vi "Verification.vi"(1 "appended array 2":string[][](array[string])) -> (0 "Array":i32[][](array[numeric]))   [LabVIEW 2019]
panel:
  in  "stop 2":bool
  in  "Blank Button 48":bool
  in  "Blank Button 47":bool
  in  "Blank Button 46":bool
  in  "Blank Button 45":bool
  in  "Blank Button 44":bool
  in  "Blank Button 43":bool
  in  "Blank Button 42":bool
  in  "Blank Button 41":bool
  in  "Color Box 45":u32(colorbox)
  in  "Color Box 46":u32(colorbox)
  in  "Color Box 48":u32(colorbox)
  in  "Color Box 43":u32(colorbox)
  in  "Color Box 41":u32(colorbox)
  in  "Color Box 42":u32(colorbox)
  in  "Color Box 44":u32(colorbox)
  in  "Color Box 47":u32(colorbox)
  in  "Blank Button 40":bool
  in  "Blank Button 39":bool
  in  "Color Box 40":u32(colorbox)
  in  "Color Box 39":u32(colorbox)
  in  "Blank Button 38":bool
  in  "Blank Button 37":bool
  in  "Color Box 38":u32(colorbox)
  in  "Color Box 37":u32(colorbox)
  in  "Blank Button 36":bool
  in  "Blank Button 35":bool
  in  "Color Box 36":u32(colorbox)
  in  "Color Box 35":u32(colorbox)
  in  "Blank Button 34":bool
  in  "Blank Button 33":bool
  in  "Color Box 34":u32(colorbox)
  in  "Color Box 33":u32(colorbox)
  in  "Blank Button 32":bool
  in  "Blank Button 31":bool
  in  "Color Box 32":u32(colorbox)
  in  "Color Box 31":u32(colorbox)
  in  "Blank Button 30":bool
  in  "Blank Button 29":bool
  in  "Color Box 30":u32(colorbox)
  in  "Color Box 29":u32(colorbox)
  in  "Blank Button 28":bool
  in  "Blank Button 27":bool
  in  "Color Box 28":u32(colorbox)
  in  "Color Box 27":u32(colorbox)
  in  "Blank Button 26":bool
  in  "Blank Button 25":bool
  in  "Color Box 26":u32(colorbox)
  in  "Color Box 25":u32(colorbox)
  in  "Blank Button 24":bool
  in  "Blank Button 23":bool
  in  "Blank Button 22":bool
  in  "Blank Button 21":bool
  in  "Blank Button 20":bool
  in  "Blank Button 19":bool
  in  "Blank Button 18":bool
  in  "Blank Button 17":bool
  in  "Color Box 24":u32(colorbox)
  in  "Color Box 22":u32(colorbox)
  in  "Color Box 21":u32(colorbox)
  in  "Color Box 19":u32(colorbox)
  in  "Color Box 23":u32(colorbox)
  in  "Color Box 18":u32(colorbox)
  in  "Color Box 17":u32(colorbox)
  in  "Color Box 20":u32(colorbox)
  in  "Blank Button 16":bool
  in  "Blank Button 15":bool
  in  "Blank Button 14":bool
  in  "Blank Button 13":bool
  in  "Blank Button 12":bool
  in  "Blank Button 11":bool
  in  "Blank Button 10":bool
  in  "Blank Button 9":bool
  in  "Color Box 16":u32(colorbox)
  in  "Color Box 14":u32(colorbox)
  in  "Color Box 11":u32(colorbox)
  in  "Color Box 13":u32(colorbox)
  in  "Color Box 9":u32(colorbox)
  in  "Color Box 15":u32(colorbox)
  in  "Color Box 12":u32(colorbox)
  in  "Color Box 10":u32(colorbox)
  in  "Blank Button 8":bool
  in  "Blank Button 7":bool
  in  "Blank Button 6":bool
  in  "Blank Button 5":bool
  in  "Blank Button 2":bool
  in  "Blank Button":bool
  in  "Color Box 2":u32(colorbox)
  in  "Color Box":u32(colorbox)
  in  "Blank Button 4":bool
  in  "Blank Button 3":bool
  in  "Color Box 4":u32(colorbox)
  in  "Color Box 3":u32(colorbox)
  in  "Color Box 8":u32(colorbox)
  in  "Color Box 5":u32(colorbox)
  in  "Color Box 6":u32(colorbox)
  in  "Color Box 7":u32(colorbox)
  in  "stop":bool
  in  "Blanc":dbl
  in  "Vert":dbl
  in  "Bleu":dbl
  in  "Orange":dbl
  in  "Jaune":dbl
  in  "Rouge":dbl
  # "Vérification des couleurs"
  # "W"
  # "R"
  # "B"
  # "G"
  # "Y"
  # "O"
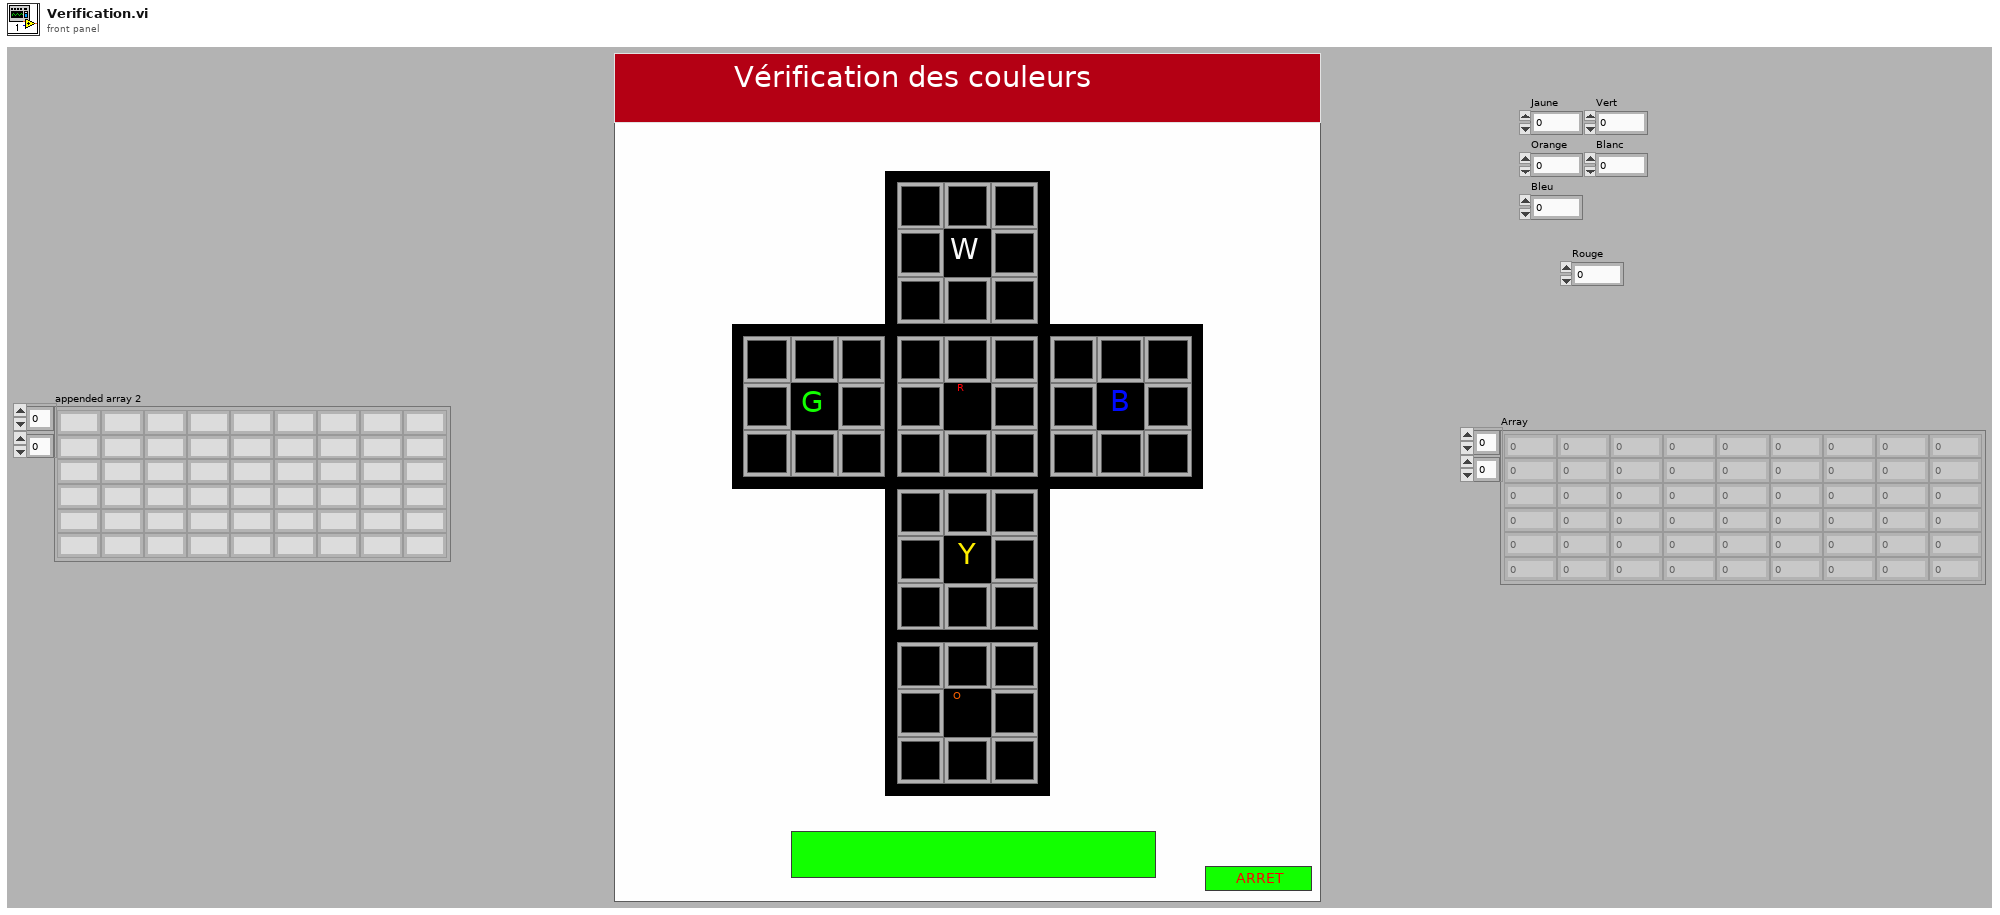
[diagram p1: front panel]
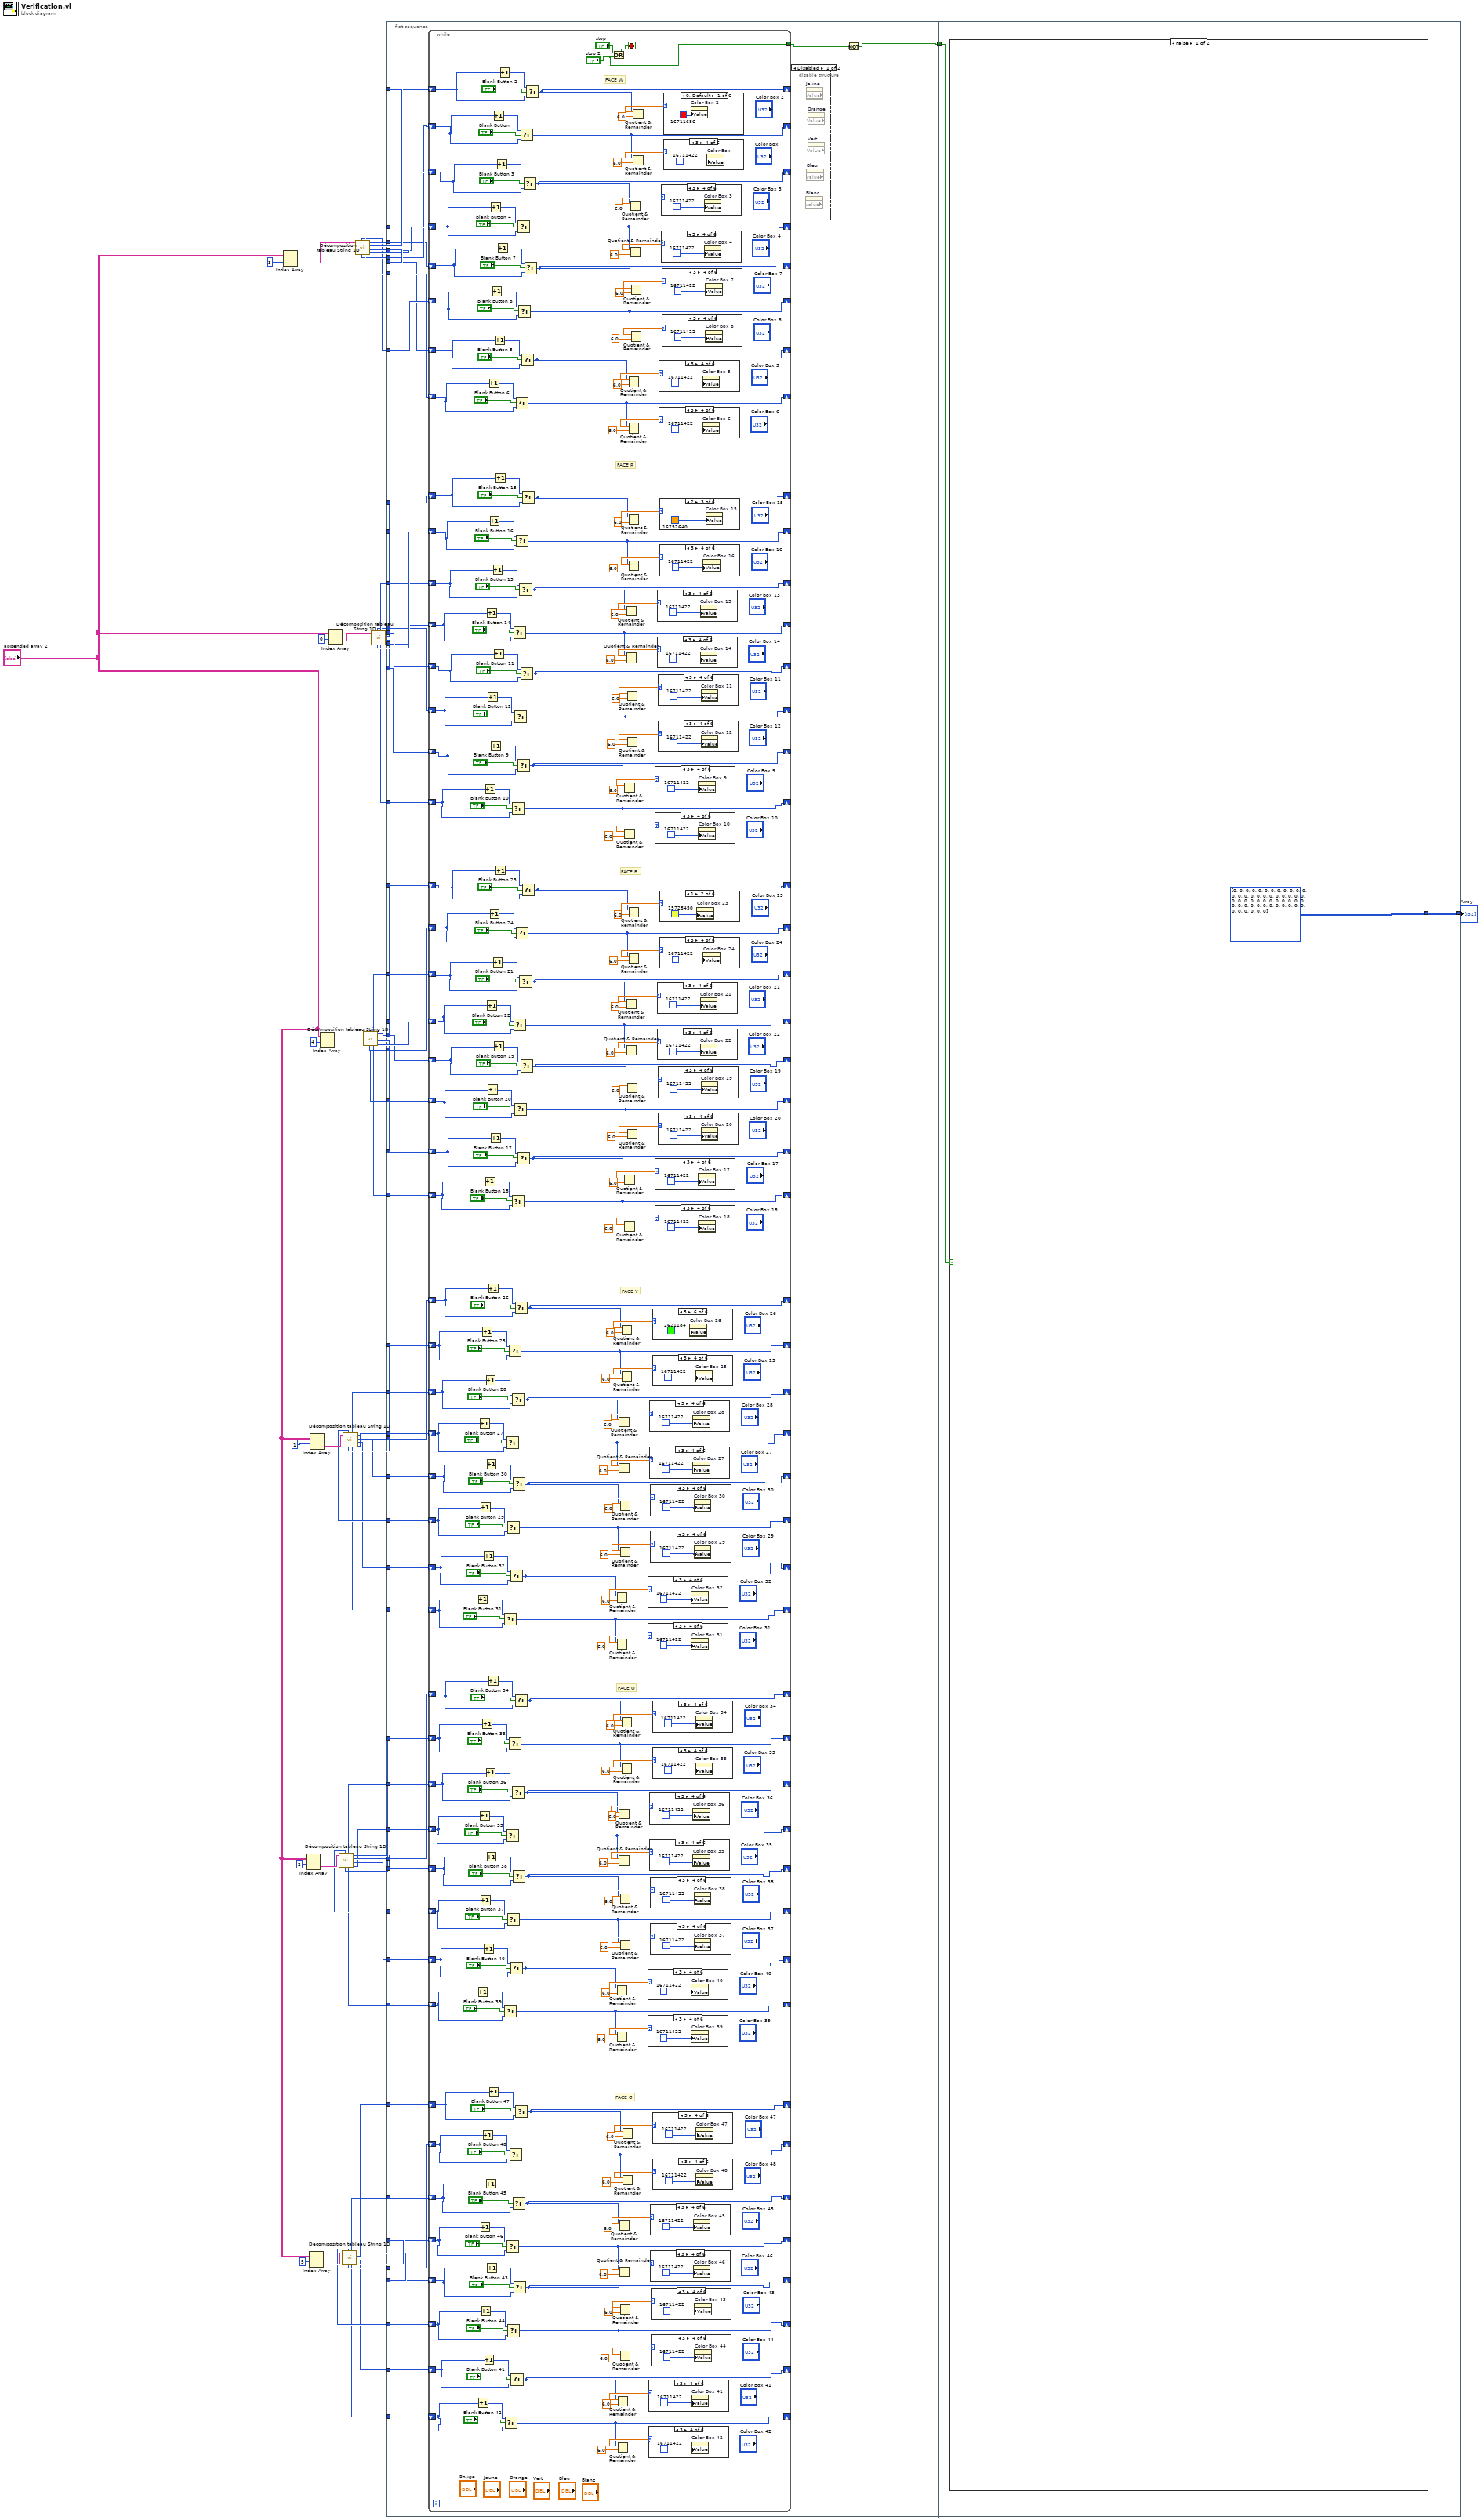
[diagram p0: block diagram]
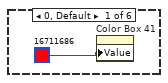
[diagram p3: hidden frame]
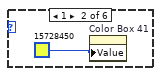
[diagram p4: hidden frame]
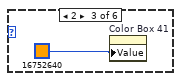
[diagram p5: hidden frame]
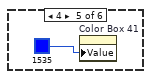
[diagram p6: hidden frame]
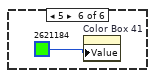
[diagram p7: hidden frame]
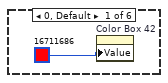
[diagram p8: hidden frame]
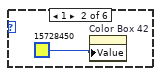
[diagram p9: hidden frame]
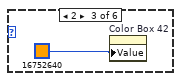
[diagram p10: hidden frame]
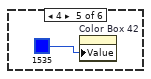
[diagram p11: hidden frame]
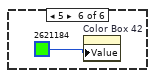
[diagram p12: hidden frame]
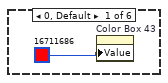
[diagram p13: hidden frame]
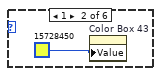
[diagram p14: hidden frame]
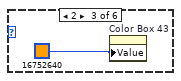
[diagram p15: hidden frame]
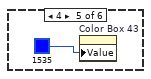
[diagram p16: hidden frame]
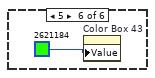
[diagram p17: hidden frame]
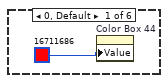
[diagram p18: hidden frame]
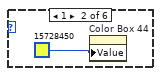
[diagram p19: hidden frame]
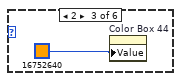
[diagram p20: hidden frame]
diagram:
  n1 = Index Array(array="appended array 2", index (row)=3) -> (element=w62:string[])  [unwired: 1 in]
  n2 = Index Array(array="appended array 2", index (row)=2) -> (element=w38:string[])  [unwired: 1 in]
  n3 = Index Array(array="appended array 2", index (row)=5) -> (element=w39:string[])  [unwired: 1 in]
  n4 = Index Array(array="appended array 2", index (row)=1) -> (element=w37:string[])  [unwired: 1 in]
  n5 = Index Array(array="appended array 2", index (row)=4) -> (element=w42:string[])  [unwired: 1 in]
  n6 = Index Array(array="appended array 2", index (row)=0) -> (element=w53:string[])  [unwired: 1 in]
  n7 = call "Décomposition tableau String 1D.vi"("appended array in"=w38) -> ("7"=w23:i32, "6"=w20:i32, "4"=w26:i32, "3"=w22:i32, "8"=w19:i32, "2"=w24:i32, "9"=w25:i32, "1"=w21:i32)  [unwired: 3 in]
  n8 = call "Décomposition tableau String 1D.vi"("appended array in"=w39) -> ("7"=w31:i32, "6"=w28:i32, "4"=w34:i32, "3"=w30:i32, "8"=w27:i32, "2"=w32:i32, "9"=w33:i32, "1"=w29:i32)  [unwired: 3 in]
  n9 = call "Décomposition tableau String 1D.vi"("appended array in"=w37) -> ("7"=w15:i32, "6"=w12:i32, "4"=w18:i32, "3"=w14:i32, "8"=w11:i32, "2"=w16:i32, "9"=w17:i32, "1"=w13:i32)  [unwired: 3 in]
  n10 = call "Décomposition tableau String 1D.vi"("appended array in"=w62) -> ("7"=w58:i32, "6"=w59:i32, "4"=w55:i32, "3"=w60:i32, "8"=w57:i32, "2"=w61:i32, "9"=w56:i32, "1"=w52:i32)  [unwired: 3 in]
  n11 = call "Décomposition tableau String 1D.vi"("appended array in"=w42) -> ("7"=w7:i32, "6"=w4:i32, "4"=w10:i32, "3"=w6:i32, "8"=w3:i32, "2"=w8:i32, "9"=w9:i32, "1"=w5:i32)  [unwired: 3 in]
  n12 = call "Décomposition tableau String 1D.vi"("appended array in"=w53) -> ("7"=w48:i32, "6"=w45:i32, "4"=w50:i32, "3"=w47:i32, "8"=w44:i32, "2"=w51:i32, "9"=w49:i32, "1"=w46:i32)  [unwired: 3 in]
  n13 = flat-sequence {
    tunnel: w61 -> [w113]
    tunnel: w60 -> [w109]
    tunnel: w58 -> [w112]
    tunnel: w57 -> [w111]
    tunnel: w56 -> [w110]
    tunnel: w55 -> [w64]
    tunnel: w52 -> [w108]
    tunnel: w59 -> [w107]
    tunnel: w44 -> [w106]
    tunnel: w46 -> [w105]
    tunnel: w50 -> [w104]
    tunnel: w49 -> [w103]
    tunnel: w47 -> [w102]
    tunnel: w48 -> [w101]
    tunnel: w51 -> [w100]
    tunnel: w45 -> [w99]
    tunnel: w34 -> [w98]
    tunnel: w33 -> [w97]
    tunnel: w32 -> [w96]
    tunnel: w31 -> [w95]
    tunnel: w30 -> [w94]
    tunnel: w29 -> [w93]
    tunnel: w28 -> [w92]
    tunnel: w27 -> [w91]
    tunnel: w26 -> [w90]
    tunnel: w25 -> [w89]
    tunnel: w24 -> [w88]
    tunnel: w23 -> [w87]
    tunnel: w22 -> [w86]
    tunnel: w21 -> [w85]
    tunnel: w20 -> [w84]
    tunnel: w19 -> [w83]
    tunnel: w18 -> [w82]
    tunnel: w17 -> [w81]
    tunnel: w16 -> [w80]
    tunnel: w15 -> [w79]
    tunnel: w14 -> [w78]
    tunnel: w13 -> [w77]
    tunnel: w12 -> [w76]
    tunnel: w11 -> [w75]
    tunnel: w10 -> [w74]
    tunnel: w9 -> [w73]
    tunnel: w8 -> [w72]
    tunnel: w7 -> [w71]
    tunnel: w6 -> [w70]
    tunnel: w5 -> [w69]
    tunnel: w4 -> [w68]
    tunnel: w3 -> [w67]
    tunnel: [w65] -> w1
    tunnel: [w694] -> w2
    tunnel: w1 -> [w693]
    frame #0 {
      n14 = while {
        shift-right: [w398] -> _
        shift-left: w64 -> [w395]
        shift-right: [w396] -> _
        shift-left: w110 -> [w402]
        shift-right: [w383] -> _
        shift-left: w113 -> [w384]
        shift-right: [w381] -> _
        shift-left: w112 -> [w382]
        shift-right: [w362] -> _
        shift-left: w109 -> [w357]
        shift-right: [w361] -> _
        shift-left: w108 -> [w358]
        shift-right: [w360] -> _
        shift-left: w107 -> [w363]
        shift-right: [w359] -> _
        shift-left: w111 -> [w364]
        shift-right: [w323] -> _
        shift-left: w104 -> [w324]
        shift-right: [w322] -> _
        shift-left: w103 -> [w315]
        shift-right: [w321] -> _
        shift-left: w100 -> [w314]
        shift-right: [w320] -> _
        shift-left: w101 -> [w313]
        shift-right: [w319] -> _
        shift-left: w102 -> [w312]
        shift-right: [w318] -> _
        shift-left: w105 -> [w311]
        shift-right: [w317] -> _
        shift-left: w99 -> [w310]
        shift-right: [w316] -> _
        shift-left: w106 -> [w309]
        shift-right: [w276] -> _
        shift-left: w74 -> [w268]
        shift-right: [w275] -> _
        shift-left: w73 -> [w267]
        shift-right: [w274] -> _
        shift-left: w72 -> [w266]
        shift-right: [w273] -> _
        shift-left: w71 -> [w265]
        shift-right: [w272] -> _
        shift-left: w70 -> [w264]
        shift-right: [w271] -> _
        shift-left: w69 -> [w263]
        shift-right: [w270] -> _
        shift-left: w68 -> [w262]
        shift-right: [w269] -> _
        shift-left: w67 -> [w261]
        shift-right: [w174] -> _
        shift-left: w82 -> [w169]
        shift-right: [w173] -> _
        shift-left: w81 -> [w170]
        shift-right: [w172] -> _
        shift-left: w80 -> [w171]
        shift-right: [w175] -> _
        shift-left: w79 -> [w168]
        shift-right: [w176] -> _
        shift-left: w78 -> [w167]
        shift-right: [w177] -> _
        shift-left: w77 -> [w166]
        shift-right: [w178] -> _
        shift-left: w76 -> [w165]
        shift-right: [w179] -> _
        shift-left: w75 -> [w180]
        shift-right: [w195] -> _
        shift-left: w90 -> [w196]
        shift-right: [w194] -> _
        shift-left: w89 -> [w187]
        shift-right: [w193] -> _
        shift-left: w88 -> [w186]
        shift-right: [w192] -> _
        shift-left: w87 -> [w183]
        shift-right: [w191] -> _
        shift-left: w86 -> [w185]
        shift-right: [w190] -> _
        shift-left: w85 -> [w184]
        shift-right: [w189] -> _
        shift-left: w84 -> [w182]
        shift-right: [w188] -> _
        shift-left: w83 -> [w181]
        shift-right: [w132] -> _
        shift-left: w98 -> [w130]
        shift-right: [w129] -> _
        shift-left: w97 -> [w131]
        shift-right: [w128] -> _
        shift-left: w96 -> [w117]
        shift-right: [w127] -> _
        shift-left: w95 -> [w118]
        shift-right: [w126] -> _
        shift-left: w94 -> [w119]
        shift-right: [w125] -> _
        shift-left: w93 -> [w120]
        shift-right: [w124] -> _
        shift-left: w92 -> [w121]
        shift-right: [w123] -> _
        shift-left: w91 -> [w122]
        tunnel: ["stop 2"] -> w66
        stop <- w116 stop-if-true
        # "FACE G"
        # "FACE O"
        # "FACE Y"
        # "FACE B"
        # "FACE R"
        # "FACE W"
        n15 = Increment(x=w180) -> (x+1=w246:i32)
        n16 = Increment(x=w181) -> (x+1=w211:i32)
        n17 = Increment(x=w122) -> (x+1=w150:i32)
        n18 = Increment(x=w168) -> (x+1=w243:i32)
        n19 = Increment(x=w183) -> (x+1=w214:i32)
        n20 = Increment(x=w118) -> (x+1=w147:i32)
        n21 = Increment(x=w166) -> (x+1=w259:i32)
        n22 = Increment(x=w184) -> (x+1=w198:i32)
        n23 = Increment(x=w120) -> (x+1=w163:i32)
        n24 = Increment(x=w170) -> (x+1=w230:i32)
        n25 = Increment(x=w187) -> (x+1=w227:i32)
        n26 = Increment(x=w131) -> (x+1=w134:i32)
        n27 = Increment(x=w165) -> (x+1=w245:i32)
        n28 = Increment(x=w182) -> (x+1=w212:i32)
        n29 = Increment(x=w121) -> (x+1=w149:i32)
        n30 = Increment(x=w309) -> (x+1=w342:i32)
        n31 = Increment(x=w261) -> (x+1=w291:i32)
        n32 = Increment(x=w171) -> (x+1=w244:i32)
        n33 = Increment(x=w186) -> (x+1=w213:i32)
        n34 = Increment(x=w117) -> (x+1=w148:i32)
        n35 = Increment(x=w167) -> (x+1=w260:i32)
        n36 = Increment(x=w185) -> (x+1=w197:i32)
        n37 = Increment(x=w313) -> (x+1=w339:i32)
        n38 = Increment(x=w265) -> (x+1=w294:i32)
        n39 = Increment(x=w119) -> (x+1=w164:i32)
        n40 = Increment(x=w311) -> (x+1=w355:i32)
        n41 = Increment(x=w263) -> (x+1=w278:i32)
        n42 = Increment(x=w169) -> (x+1=w229:i32)
        n43 = Increment(x=w196) -> (x+1=w228:i32)
        n44 = Increment(x=w130) -> (x+1=w133:i32)
        n45 = Increment(x=w364) -> (x+1=w379:i32)
        n46 = Increment(x=w315) -> (x+1=w326:i32)
        n47 = Increment(x=w267) -> (x+1=w307:i32)
        n48 = Increment(x=w382) -> (x+1=w386:i32)
        n49 = Increment(x=w310) -> (x+1=w341:i32)
        n50 = Increment(x=w262) -> (x+1=w292:i32)
        n51 = Increment(x=w358) -> (x+1=w366:i32)
        n52 = Increment(x=w314) -> (x+1=w340:i32)
        n53 = Increment(x=w266) -> (x+1=w293:i32)
        n54 = Increment(x=w402) -> (x+1=w403:i32)
        n55 = Increment(x=w312) -> (x+1=w356:i32)
        n56 = Increment(x=w264) -> (x+1=w277:i32)
        n57 = Increment(x=w363) -> (x+1=w380:i32)
        n58 = Increment(x=w324) -> (x+1=w325:i32)
        n59 = Increment(x=w268) -> (x+1=w308:i32)
        n60 = Increment(x=w384) -> (x+1=w385:i32)
        n61 = Increment(x=w357) -> (x+1=w365:i32)
        n62 = Increment(x=w395) -> (x+1=w404:i32)
        n63 = Select(t=w246, s="Blank Button 31", f=w180) -> (s? t:f=w179:i32)
        n64 = Select(t=w211, s="Blank Button 39", f=w181) -> (s? t:f=w188:i32)
        n65 = Select(t=w150, s="Blank Button 42", f=w122) -> (s? t:f=w123:i32)
        n66 = Select(t=w243, s="Blank Button 27", f=w168) -> (s? t:f=w175:i32)
        n67 = Select(t=w214, s="Blank Button 35", f=w183) -> (s? t:f=w192:i32)
        n68 = Select(t=w147, s="Blank Button 46", f=w118) -> (s? t:f=w127:i32)
        n69 = Select(t=w259, s="Blank Button 29", f=w166) -> (s? t:f=w177:i32)
        n70 = Select(t=w198, s="Blank Button 37", f=w184) -> (s? t:f=w190:i32)
        n71 = Select(t=w163, s="Blank Button 44", f=w120) -> (s? t:f=w125:i32)
        n72 = Select(t=w230, s="Blank Button 25", f=w170) -> (s? t:f=w173:i32)
        n73 = Select(t=w227, s="Blank Button 33", f=w187) -> (s? t:f=w194:i32)
        n74 = Select(t=w134, s="Blank Button 48", f=w131) -> (s? t:f=w129:i32)
        n75 = Select(t=w245, s="Blank Button 32", f=w165) -> (s? t:f=w178:i32)
        n76 = Select(t=w212, s="Blank Button 40", f=w182) -> (s? t:f=w189:i32)
        n77 = Select(t=w149, s="Blank Button 41", f=w121) -> (s? t:f=w124:i32)
        n78 = Select(t=w342, s="Blank Button 10", f=w309) -> (s? t:f=w316:i32)
        n79 = Select(t=w291, s="Blank Button 18", f=w261) -> (s? t:f=w269:i32)
        n80 = Select(t=w244, s="Blank Button 28", f=w171) -> (s? t:f=w172:i32)
        n81 = Select(t=w213, s="Blank Button 36", f=w186) -> (s? t:f=w193:i32)
        n82 = Select(t=w148, s="Blank Button 45", f=w117) -> (s? t:f=w128:i32)
        n83 = Select(t=w260, s="Blank Button 30", f=w167) -> (s? t:f=w176:i32)
        n84 = Select(t=w197, s="Blank Button 38", f=w185) -> (s? t:f=w191:i32)
        n85 = Select(t=w339, s="Blank Button 14", f=w313) -> (s? t:f=w320:i32)
        n86 = Select(t=w294, s="Blank Button 22", f=w265) -> (s? t:f=w273:i32)
        n87 = Select(t=w164, s="Blank Button 43", f=w119) -> (s? t:f=w126:i32)
        n88 = Select(t=w355, s="Blank Button 12", f=w311) -> (s? t:f=w318:i32)
        n89 = Select(t=w278, s="Blank Button 20", f=w263) -> (s? t:f=w271:i32)
        n90 = Select(t=w229, s="Blank Button 26", f=w169) -> (s? t:f=w174:i32)
        n91 = Select(t=w228, s="Blank Button 34", f=w196) -> (s? t:f=w195:i32)
        n92 = Select(t=w133, s="Blank Button 47", f=w130) -> (s? t:f=w132:i32)
        n93 = Select(t=w379, s="Blank Button 6", f=w364) -> (s? t:f=w359:i32)
        n94 = Select(t=w326, s="Blank Button 16", f=w315) -> (s? t:f=w322:i32)
        n95 = Select(t=w307, s="Blank Button 24", f=w267) -> (s? t:f=w275:i32)
        n96 = Select(t=w386, s="Blank Button 4", f=w382) -> (s? t:f=w381:i32)
        n97 = Select(t=w341, s="Blank Button 9", f=w310) -> (s? t:f=w317:i32)
        n98 = Select(t=w292, s="Blank Button 17", f=w262) -> (s? t:f=w270:i32)
        n99 = Select(t=w366, s="Blank Button 8", f=w358) -> (s? t:f=w361:i32)
        n100 = Select(t=w340, s="Blank Button 13", f=w314) -> (s? t:f=w321:i32)
        n101 = Select(t=w293, s="Blank Button 21", f=w266) -> (s? t:f=w274:i32)
        n102 = Select(t=w403, s="Blank Button", f=w402) -> (s? t:f=w396:i32)
        n103 = Select(t=w356, s="Blank Button 11", f=w312) -> (s? t:f=w319:i32)
        n104 = Select(t=w277, s="Blank Button 19", f=w264) -> (s? t:f=w272:i32)
        n105 = Select(t=w380, s="Blank Button 5", f=w363) -> (s? t:f=w360:i32)
        n106 = Select(t=w325, s="Blank Button 15", f=w324) -> (s? t:f=w323:i32)
        n107 = Select(t=w308, s="Blank Button 23", f=w268) -> (s? t:f=w276:i32)
        n108 = Select(t=w385, s="Blank Button 3", f=w384) -> (s? t:f=w383:i32)
        n109 = Select(t=w365, s="Blank Button 7", f=w357) -> (s? t:f=w362:i32)
        n110 = Select(t=w404, s="Blank Button 2", f=w395) -> (s? t:f=w398:i32)
        n111 = Or(x="stop", y="stop 2") -> (x .or. y?=w116:bool)
        n112 = Quotient & Remainder(x=w178, y=6.0) -> (x-y*floor(x/y)=w249:dbl)  [unwired: 1 out]
        n113 = Quotient & Remainder(x=w179, y=6.0) -> (x-y*floor(x/y)=w247:dbl)  [unwired: 1 out]
        n114 = Quotient & Remainder(x=w189, y=6.0) -> (x-y*floor(x/y)=w208:dbl)  [unwired: 1 out]
        n115 = Quotient & Remainder(x=w188, y=6.0) -> (x-y*floor(x/y)=w210:dbl)  [unwired: 1 out]
        n116 = Quotient & Remainder(x=w124, y=6.0) -> (x-y*floor(x/y)=w153:dbl)  [unwired: 1 out]
        n117 = Quotient & Remainder(x=w123, y=6.0) -> (x-y*floor(x/y)=w151:dbl)  [unwired: 1 out]
        n118 = Quotient & Remainder(x=w172, y=6.0) -> (x-y*floor(x/y)=w240:dbl)  [unwired: 1 out]
        n119 = Quotient & Remainder(x=w175, y=6.0) -> (x-y*floor(x/y)=w242:dbl)  [unwired: 1 out]
        n120 = Quotient & Remainder(x=w193, y=6.0) -> (x-y*floor(x/y)=w217:dbl)  [unwired: 1 out]
        n121 = Quotient & Remainder(x=w192, y=6.0) -> (x-y*floor(x/y)=w215:dbl)  [unwired: 1 out]
        n122 = Quotient & Remainder(x=w128, y=6.0) -> (x-y*floor(x/y)=w144:dbl)  [unwired: 1 out]
        n123 = Quotient & Remainder(x=w127, y=6.0) -> (x-y*floor(x/y)=w146:dbl)  [unwired: 1 out]
        n124 = Quotient & Remainder(x=w176, y=6.0) -> (x-y*floor(x/y)=w256:dbl)  [unwired: 1 out]
        n125 = Quotient & Remainder(x=w177, y=6.0) -> (x-y*floor(x/y)=w258:dbl)  [unwired: 1 out]
        n126 = Quotient & Remainder(x=w191, y=6.0) -> (x-y*floor(x/y)=w201:dbl)  [unwired: 1 out]
        n127 = Quotient & Remainder(x=w190, y=6.0) -> (x-y*floor(x/y)=w199:dbl)  [unwired: 1 out]
        n128 = Quotient & Remainder(x=w126, y=6.0) -> (x-y*floor(x/y)=w160:dbl)  [unwired: 1 out]
        n129 = Quotient & Remainder(x=w125, y=6.0) -> (x-y*floor(x/y)=w162:dbl)  [unwired: 1 out]
        n130 = Quotient & Remainder(x=w174, y=6.0) -> (x-y*floor(x/y)=w233:dbl)  [unwired: 1 out]
        n131 = Quotient & Remainder(x=w173, y=6.0) -> (x-y*floor(x/y)=w231:dbl)  [unwired: 1 out]
        n132 = Quotient & Remainder(x=w195, y=6.0) -> (x-y*floor(x/y)=w224:dbl)  [unwired: 1 out]
        n133 = Quotient & Remainder(x=w194, y=6.0) -> (x-y*floor(x/y)=w226:dbl)  [unwired: 1 out]
        n134 = Quotient & Remainder(x=w132, y=6.0) -> (x-y*floor(x/y)=w137:dbl)  [unwired: 1 out]
        n135 = Quotient & Remainder(x=w129, y=6.0) -> (x-y*floor(x/y)=w135:dbl)  [unwired: 1 out]
        n136 = Quotient & Remainder(x=w317, y=6.0) -> (x-y*floor(x/y)=w345:dbl)  [unwired: 1 out]
        n137 = Quotient & Remainder(x=w316, y=6.0) -> (x-y*floor(x/y)=w343:dbl)  [unwired: 1 out]
        n138 = Quotient & Remainder(x=w270, y=6.0) -> (x-y*floor(x/y)=w288:dbl)  [unwired: 1 out]
        n139 = Quotient & Remainder(x=w269, y=6.0) -> (x-y*floor(x/y)=w290:dbl)  [unwired: 1 out]
        n140 = Quotient & Remainder(x=w321, y=6.0) -> (x-y*floor(x/y)=w336:dbl)  [unwired: 1 out]
        n141 = Quotient & Remainder(x=w320, y=6.0) -> (x-y*floor(x/y)=w338:dbl)  [unwired: 1 out]
        n142 = Quotient & Remainder(x=w274, y=6.0) -> (x-y*floor(x/y)=w297:dbl)  [unwired: 1 out]
        n143 = Quotient & Remainder(x=w273, y=6.0) -> (x-y*floor(x/y)=w295:dbl)  [unwired: 1 out]
        n144 = Quotient & Remainder(x=w319, y=6.0) -> (x-y*floor(x/y)=w352:dbl)  [unwired: 1 out]
        n145 = Quotient & Remainder(x=w318, y=6.0) -> (x-y*floor(x/y)=w354:dbl)  [unwired: 1 out]
        n146 = Quotient & Remainder(x=w272, y=6.0) -> (x-y*floor(x/y)=w281:dbl)  [unwired: 1 out]
        n147 = Quotient & Remainder(x=w271, y=6.0) -> (x-y*floor(x/y)=w279:dbl)  [unwired: 1 out]
        n148 = Quotient & Remainder(x=w360, y=6.0) -> (x-y*floor(x/y)=w376:dbl)  [unwired: 1 out]
        n149 = Quotient & Remainder(x=w359, y=6.0) -> (x-y*floor(x/y)=w378:dbl)  [unwired: 1 out]
        n150 = Quotient & Remainder(x=w323, y=6.0) -> (x-y*floor(x/y)=w329:dbl)  [unwired: 1 out]
        n151 = Quotient & Remainder(x=w322, y=6.0) -> (x-y*floor(x/y)=w327:dbl)  [unwired: 1 out]
        n152 = Quotient & Remainder(x=w276, y=6.0) -> (x-y*floor(x/y)=w304:dbl)  [unwired: 1 out]
        n153 = Quotient & Remainder(x=w275, y=6.0) -> (x-y*floor(x/y)=w306:dbl)  [unwired: 1 out]
        n154 = Quotient & Remainder(x=w383, y=6.0) -> (x-y*floor(x/y)=w389:dbl)  [unwired: 1 out]
        n155 = Quotient & Remainder(x=w381, y=6.0) -> (x-y*floor(x/y)=w387:dbl)  [unwired: 1 out]
        n156 = Quotient & Remainder(x=w362, y=6.0) -> (x-y*floor(x/y)=w369:dbl)  [unwired: 1 out]
        n157 = Quotient & Remainder(x=w361, y=6.0) -> (x-y*floor(x/y)=w367:dbl)  [unwired: 1 out]
        n158 = Quotient & Remainder(x=w398, y=6.0) -> (x-y*floor(x/y)=w399:dbl)  [unwired: 1 out]
        n159 = Quotient & Remainder(x=w396, y=6.0) -> (x-y*floor(x/y)=w401:dbl)  [unwired: 1 out]
        n160 = case shown="3" w249 {
          frame 0, Default {
            n161 = property on="Color Box 32" class="ColBox"("Value"=u32 16711686 ("Color Box")) -> ()  [unwired: 2 in, 2 out]
          }
          frame 1 {
            n162 = property on="Color Box 32" class="ColBox"("Value"=u32 15728450 ("Color Box")) -> ()  [unwired: 2 in, 2 out]
          }
          frame 2 {
            n163 = property on="Color Box 32" class="ColBox"("Value"=u32 16752640 ("Color Box")) -> ()  [unwired: 2 in, 2 out]
          }
          frame 3 {
            n164 = property on="Color Box 32" class="ColBox"("Value"=u32 16711422 ("Color Box")) -> ()  [unwired: 2 in, 2 out]
          }
          frame 4 {
            n165 = property on="Color Box 32" class="ColBox"("Value"=u32 1535 ("Color Box")) -> ()  [unwired: 2 in, 2 out]
          }
          frame 5 {
            n166 = property on="Color Box 32" class="ColBox"("Value"=u32 2621184 ("Color Box")) -> ()  [unwired: 2 in, 2 out]
          }
        }
        n167 = case shown="3" w247 {
          frame 0, Default {
            n168 = property on="Color Box 31" class="ColBox"("Value"=u32 16711686 ("Color Box")) -> ()  [unwired: 2 in, 2 out]
          }
          frame 1 {
            n169 = property on="Color Box 31" class="ColBox"("Value"=u32 15728450 ("Color Box")) -> ()  [unwired: 2 in, 2 out]
          }
          frame 2 {
            n170 = property on="Color Box 31" class="ColBox"("Value"=u32 16752640 ("Color Box")) -> ()  [unwired: 2 in, 2 out]
          }
          frame 3 {
            n171 = property on="Color Box 31" class="ColBox"("Value"=u32 16711422 ("Color Box")) -> ()  [unwired: 2 in, 2 out]
          }
          frame 4 {
            n172 = property on="Color Box 31" class="ColBox"("Value"=u32 1535 ("Color Box")) -> ()  [unwired: 2 in, 2 out]
          }
          frame 5 {
            n173 = property on="Color Box 31" class="ColBox"("Value"=u32 2621184 ("Color Box")) -> ()  [unwired: 2 in, 2 out]
          }
        }
        n174 = case shown="3" w208 {
          frame 0, Default {
            n175 = property on="Color Box 40" class="ColBox"("Value"=u32 16711686 ("Color Box")) -> ()  [unwired: 2 in, 2 out]
          }
          frame 1 {
            n176 = property on="Color Box 40" class="ColBox"("Value"=u32 15728450 ("Color Box")) -> ()  [unwired: 2 in, 2 out]
          }
          frame 2 {
            n177 = property on="Color Box 40" class="ColBox"("Value"=u32 16752640 ("Color Box")) -> ()  [unwired: 2 in, 2 out]
          }
          frame 3 {
            n178 = property on="Color Box 40" class="ColBox"("Value"=u32 16711422 ("Color Box")) -> ()  [unwired: 2 in, 2 out]
          }
          frame 4 {
            n179 = property on="Color Box 40" class="ColBox"("Value"=u32 1535 ("Color Box")) -> ()  [unwired: 2 in, 2 out]
          }
          frame 5 {
            n180 = property on="Color Box 40" class="ColBox"("Value"=u32 2621184 ("Color Box")) -> ()  [unwired: 2 in, 2 out]
          }
        }
        n181 = case shown="3" w210 {
          frame 0, Default {
            n182 = property on="Color Box 39" class="ColBox"("Value"=u32 16711686 ("Color Box")) -> ()  [unwired: 2 in, 2 out]
          }
          frame 1 {
            n183 = property on="Color Box 39" class="ColBox"("Value"=u32 15728450 ("Color Box")) -> ()  [unwired: 2 in, 2 out]
          }
          frame 2 {
            n184 = property on="Color Box 39" class="ColBox"("Value"=u32 16752640 ("Color Box")) -> ()  [unwired: 2 in, 2 out]
          }
          frame 3 {
            n185 = property on="Color Box 39" class="ColBox"("Value"=u32 16711422 ("Color Box")) -> ()  [unwired: 2 in, 2 out]
          }
          frame 4 {
            n186 = property on="Color Box 39" class="ColBox"("Value"=u32 1535 ("Color Box")) -> ()  [unwired: 2 in, 2 out]
          }
          frame 5 {
            n187 = property on="Color Box 39" class="ColBox"("Value"=u32 2621184 ("Color Box")) -> ()  [unwired: 2 in, 2 out]
          }
        }
        n188 = case shown="3" w153 {
          frame 0, Default {
            n189 = property on="Color Box 41" class="ColBox"("Value"=u32 16711686 ("Color Box")) -> ()  [unwired: 2 in, 2 out]
          }
          frame 1 {
            n190 = property on="Color Box 41" class="ColBox"("Value"=u32 15728450 ("Color Box")) -> ()  [unwired: 2 in, 2 out]
          }
          frame 2 {
            n191 = property on="Color Box 41" class="ColBox"("Value"=u32 16752640 ("Color Box")) -> ()  [unwired: 2 in, 2 out]
          }
          frame 3 {
            n192 = property on="Color Box 41" class="ColBox"("Value"=u32 16711422 ("Color Box")) -> ()  [unwired: 2 in, 2 out]
          }
          frame 4 {
            n193 = property on="Color Box 41" class="ColBox"("Value"=u32 1535 ("Color Box")) -> ()  [unwired: 2 in, 2 out]
          }
          frame 5 {
            n194 = property on="Color Box 41" class="ColBox"("Value"=u32 2621184 ("Color Box")) -> ()  [unwired: 2 in, 2 out]
          }
        }
        n195 = case shown="3" w151 {
          frame 0, Default {
            n196 = property on="Color Box 42" class="ColBox"("Value"=u32 16711686 ("Color Box")) -> ()  [unwired: 2 in, 2 out]
          }
          frame 1 {
            n197 = property on="Color Box 42" class="ColBox"("Value"=u32 15728450 ("Color Box")) -> ()  [unwired: 2 in, 2 out]
          }
          frame 2 {
            n198 = property on="Color Box 42" class="ColBox"("Value"=u32 16752640 ("Color Box")) -> ()  [unwired: 2 in, 2 out]
          }
          frame 3 {
            n199 = property on="Color Box 42" class="ColBox"("Value"=u32 16711422 ("Color Box")) -> ()  [unwired: 2 in, 2 out]
          }
          frame 4 {
            n200 = property on="Color Box 42" class="ColBox"("Value"=u32 1535 ("Color Box")) -> ()  [unwired: 2 in, 2 out]
          }
          frame 5 {
            n201 = property on="Color Box 42" class="ColBox"("Value"=u32 2621184 ("Color Box")) -> ()  [unwired: 2 in, 2 out]
          }
        }
        n202 = case shown="3" w240 {
          frame 0, Default {
            n203 = property on="Color Box 28" class="ColBox"("Value"=u32 16711686 ("Color Box")) -> ()  [unwired: 2 in, 2 out]
          }
          frame 1 {
            n204 = property on="Color Box 28" class="ColBox"("Value"=u32 15728450 ("Color Box")) -> ()  [unwired: 2 in, 2 out]
          }
          frame 2 {
            n205 = property on="Color Box 28" class="ColBox"("Value"=u32 16752640 ("Color Box")) -> ()  [unwired: 2 in, 2 out]
          }
          frame 3 {
            n206 = property on="Color Box 28" class="ColBox"("Value"=u32 16711422 ("Color Box")) -> ()  [unwired: 2 in, 2 out]
          }
          frame 4 {
            n207 = property on="Color Box 28" class="ColBox"("Value"=u32 1535 ("Color Box")) -> ()  [unwired: 2 in, 2 out]
          }
          frame 5 {
            n208 = property on="Color Box 28" class="ColBox"("Value"=u32 2621184 ("Color Box")) -> ()  [unwired: 2 in, 2 out]
          }
        }
        n209 = case shown="3" w242 {
          frame 0, Default {
            n210 = property on="Color Box 27" class="ColBox"("Value"=u32 16711686 ("Color Box")) -> ()  [unwired: 2 in, 2 out]
          }
          frame 1 {
            n211 = property on="Color Box 27" class="ColBox"("Value"=u32 15728450 ("Color Box")) -> ()  [unwired: 2 in, 2 out]
          }
          frame 2 {
            n212 = property on="Color Box 27" class="ColBox"("Value"=u32 16752640 ("Color Box")) -> ()  [unwired: 2 in, 2 out]
          }
          frame 3 {
            n213 = property on="Color Box 27" class="ColBox"("Value"=u32 16711422 ("Color Box")) -> ()  [unwired: 2 in, 2 out]
          }
          frame 4 {
            n214 = property on="Color Box 27" class="ColBox"("Value"=u32 1535 ("Color Box")) -> ()  [unwired: 2 in, 2 out]
          }
          frame 5 {
            n215 = property on="Color Box 27" class="ColBox"("Value"=u32 2621184 ("Color Box")) -> ()  [unwired: 2 in, 2 out]
          }
        }
        n216 = case shown="3" w217 {
          frame 0, Default {
            n217 = property on="Color Box 36" class="ColBox"("Value"=u32 16711686 ("Color Box")) -> ()  [unwired: 2 in, 2 out]
          }
          frame 1 {
            n218 = property on="Color Box 36" class="ColBox"("Value"=u32 15728450 ("Color Box")) -> ()  [unwired: 2 in, 2 out]
          }
          frame 2 {
            n219 = property on="Color Box 36" class="ColBox"("Value"=u32 16752640 ("Color Box")) -> ()  [unwired: 2 in, 2 out]
          }
          frame 3 {
            n220 = property on="Color Box 36" class="ColBox"("Value"=u32 16711422 ("Color Box")) -> ()  [unwired: 2 in, 2 out]
          }
          frame 4 {
            n221 = property on="Color Box 36" class="ColBox"("Value"=u32 1535 ("Color Box")) -> ()  [unwired: 2 in, 2 out]
          }
          frame 5 {
            n222 = property on="Color Box 36" class="ColBox"("Value"=u32 2621184 ("Color Box")) -> ()  [unwired: 2 in, 2 out]
          }
        }
        n223 = case shown="3" w215 {
          frame 0, Default {
            n224 = property on="Color Box 35" class="ColBox"("Value"=u32 16711686 ("Color Box")) -> ()  [unwired: 2 in, 2 out]
          }
          frame 1 {
            n225 = property on="Color Box 35" class="ColBox"("Value"=u32 15728450 ("Color Box")) -> ()  [unwired: 2 in, 2 out]
          }
          frame 2 {
            n226 = property on="Color Box 35" class="ColBox"("Value"=u32 16752640 ("Color Box")) -> ()  [unwired: 2 in, 2 out]
          }
          frame 3 {
            n227 = property on="Color Box 35" class="ColBox"("Value"=u32 16711422 ("Color Box")) -> ()  [unwired: 2 in, 2 out]
          }
          frame 4 {
            n228 = property on="Color Box 35" class="ColBox"("Value"=u32 1535 ("Color Box")) -> ()  [unwired: 2 in, 2 out]
          }
          frame 5 {
            n229 = property on="Color Box 35" class="ColBox"("Value"=u32 2621184 ("Color Box")) -> ()  [unwired: 2 in, 2 out]
          }
        }
        n230 = case shown="3" w144 {
          frame 0, Default {
            n231 = property on="Color Box 45" class="ColBox"("Value"=u32 16711686 ("Color Box")) -> ()  [unwired: 2 in, 2 out]
          }
          frame 1 {
            n232 = property on="Color Box 45" class="ColBox"("Value"=u32 15728450 ("Color Box")) -> ()  [unwired: 2 in, 2 out]
          }
          frame 2 {
            n233 = property on="Color Box 45" class="ColBox"("Value"=u32 16752640 ("Color Box")) -> ()  [unwired: 2 in, 2 out]
          }
          frame 3 {
            n234 = property on="Color Box 45" class="ColBox"("Value"=u32 16711422 ("Color Box")) -> ()  [unwired: 2 in, 2 out]
          }
          frame 4 {
            n235 = property on="Color Box 45" class="ColBox"("Value"=u32 1535 ("Color Box")) -> ()  [unwired: 2 in, 2 out]
          }
          frame 5 {
            n236 = property on="Color Box 45" class="ColBox"("Value"=u32 2621184 ("Color Box")) -> ()  [unwired: 2 in, 2 out]
          }
        }
        n237 = case shown="3" w146 {
          frame 0, Default {
            n238 = property on="Color Box 46" class="ColBox"("Value"=u32 16711686 ("Color Box")) -> ()  [unwired: 2 in, 2 out]
          }
          frame 1 {
            n239 = property on="Color Box 46" class="ColBox"("Value"=u32 15728450 ("Color Box")) -> ()  [unwired: 2 in, 2 out]
          }
          frame 2 {
            n240 = property on="Color Box 46" class="ColBox"("Value"=u32 16752640 ("Color Box")) -> ()  [unwired: 2 in, 2 out]
          }
          frame 3 {
            n241 = property on="Color Box 46" class="ColBox"("Value"=u32 16711422 ("Color Box")) -> ()  [unwired: 2 in, 2 out]
          }
          frame 4 {
            n242 = property on="Color Box 46" class="ColBox"("Value"=u32 1535 ("Color Box")) -> ()  [unwired: 2 in, 2 out]
          }
          frame 5 {
            n243 = property on="Color Box 46" class="ColBox"("Value"=u32 2621184 ("Color Box")) -> ()  [unwired: 2 in, 2 out]
          }
        }
        n244 = case shown="3" w256 {
          frame 0, Default {
            n245 = property on="Color Box 30" class="ColBox"("Value"=u32 16711686 ("Color Box")) -> ()  [unwired: 2 in, 2 out]
          }
          frame 1 {
            n246 = property on="Color Box 30" class="ColBox"("Value"=u32 15728450 ("Color Box")) -> ()  [unwired: 2 in, 2 out]
          }
          frame 2 {
            n247 = property on="Color Box 30" class="ColBox"("Value"=u32 16752640 ("Color Box")) -> ()  [unwired: 2 in, 2 out]
          }
          frame 3 {
            n248 = property on="Color Box 30" class="ColBox"("Value"=u32 16711422 ("Color Box")) -> ()  [unwired: 2 in, 2 out]
          }
          frame 4 {
            n249 = property on="Color Box 30" class="ColBox"("Value"=u32 1535 ("Color Box")) -> ()  [unwired: 2 in, 2 out]
          }
          frame 5 {
            n250 = property on="Color Box 30" class="ColBox"("Value"=u32 2621184 ("Color Box")) -> ()  [unwired: 2 in, 2 out]
          }
        }
        n251 = case shown="3" w258 {
          frame 0, Default {
            n252 = property on="Color Box 29" class="ColBox"("Value"=u32 16711686 ("Color Box")) -> ()  [unwired: 2 in, 2 out]
          }
          frame 1 {
            n253 = property on="Color Box 29" class="ColBox"("Value"=u32 15728450 ("Color Box")) -> ()  [unwired: 2 in, 2 out]
          }
          frame 2 {
            n254 = property on="Color Box 29" class="ColBox"("Value"=u32 16752640 ("Color Box")) -> ()  [unwired: 2 in, 2 out]
          }
          frame 3 {
            n255 = property on="Color Box 29" class="ColBox"("Value"=u32 16711422 ("Color Box")) -> ()  [unwired: 2 in, 2 out]
          }
          frame 4 {
            n256 = property on="Color Box 29" class="ColBox"("Value"=u32 1535 ("Color Box")) -> ()  [unwired: 2 in, 2 out]
          }
          frame 5 {
            n257 = property on="Color Box 29" class="ColBox"("Value"=u32 2621184 ("Color Box")) -> ()  [unwired: 2 in, 2 out]
          }
        }
        n258 = case shown="3" w201 {
          frame 0, Default {
            n259 = property on="Color Box 38" class="ColBox"("Value"=u32 16711686 ("Color Box")) -> ()  [unwired: 2 in, 2 out]
          }
          frame 1 {
            n260 = property on="Color Box 38" class="ColBox"("Value"=u32 15728450 ("Color Box")) -> ()  [unwired: 2 in, 2 out]
          }
          frame 2 {
            n261 = property on="Color Box 38" class="ColBox"("Value"=u32 16752640 ("Color Box")) -> ()  [unwired: 2 in, 2 out]
          }
          frame 3 {
            n262 = property on="Color Box 38" class="ColBox"("Value"=u32 16711422 ("Color Box")) -> ()  [unwired: 2 in, 2 out]
          }
          frame 4 {
            n263 = property on="Color Box 38" class="ColBox"("Value"=u32 1535 ("Color Box")) -> ()  [unwired: 2 in, 2 out]
          }
          frame 5 {
            n264 = property on="Color Box 38" class="ColBox"("Value"=u32 2621184 ("Color Box")) -> ()  [unwired: 2 in, 2 out]
          }
        }
        n265 = case shown="3" w199 {
          frame 0, Default {
            n266 = property on="Color Box 37" class="ColBox"("Value"=u32 16711686 ("Color Box")) -> ()  [unwired: 2 in, 2 out]
          }
          frame 1 {
            n267 = property on="Color Box 37" class="ColBox"("Value"=u32 15728450 ("Color Box")) -> ()  [unwired: 2 in, 2 out]
          }
          frame 2 {
            n268 = property on="Color Box 37" class="ColBox"("Value"=u32 16752640 ("Color Box")) -> ()  [unwired: 2 in, 2 out]
          }
          frame 3 {
            n269 = property on="Color Box 37" class="ColBox"("Value"=u32 16711422 ("Color Box")) -> ()  [unwired: 2 in, 2 out]
          }
          frame 4 {
            n270 = property on="Color Box 37" class="ColBox"("Value"=u32 1535 ("Color Box")) -> ()  [unwired: 2 in, 2 out]
          }
          frame 5 {
            n271 = property on="Color Box 37" class="ColBox"("Value"=u32 2621184 ("Color Box")) -> ()  [unwired: 2 in, 2 out]
          }
        }
        n272 = case shown="3" w160 {
          frame 0, Default {
            n273 = property on="Color Box 43" class="ColBox"("Value"=u32 16711686 ("Color Box")) -> ()  [unwired: 2 in, 2 out]
          }
          frame 1 {
            n274 = property on="Color Box 43" class="ColBox"("Value"=u32 15728450 ("Color Box")) -> ()  [unwired: 2 in, 2 out]
          }
          frame 2 {
            n275 = property on="Color Box 43" class="ColBox"("Value"=u32 16752640 ("Color Box")) -> ()  [unwired: 2 in, 2 out]
          }
          frame 3 {
            n276 = property on="Color Box 43" class="ColBox"("Value"=u32 16711422 ("Color Box")) -> ()  [unwired: 2 in, 2 out]
          }
          frame 4 {
            n277 = property on="Color Box 43" class="ColBox"("Value"=u32 1535 ("Color Box")) -> ()  [unwired: 2 in, 2 out]
          }
          frame 5 {
            n278 = property on="Color Box 43" class="ColBox"("Value"=u32 2621184 ("Color Box")) -> ()  [unwired: 2 in, 2 out]
          }
        }
        n279 = case shown="3" w162 {
          frame 0, Default {
            n280 = property on="Color Box 44" class="ColBox"("Value"=u32 16711686 ("Color Box")) -> ()  [unwired: 2 in, 2 out]
          }
          frame 1 {
            n281 = property on="Color Box 44" class="ColBox"("Value"=u32 15728450 ("Color Box")) -> ()  [unwired: 2 in, 2 out]
          }
          frame 2 {
            n282 = property on="Color Box 44" class="ColBox"("Value"=u32 16752640 ("Color Box")) -> ()  [unwired: 2 in, 2 out]
          }
          frame 3 {
            n283 = property on="Color Box 44" class="ColBox"("Value"=u32 16711422 ("Color Box")) -> ()  [unwired: 2 in, 2 out]
          }
          frame 4 {
            n284 = property on="Color Box 44" class="ColBox"("Value"=u32 1535 ("Color Box")) -> ()  [unwired: 2 in, 2 out]
          }
          frame 5 {
            n285 = property on="Color Box 44" class="ColBox"("Value"=u32 2621184 ("Color Box")) -> ()  [unwired: 2 in, 2 out]
          }
        }
        n286 = case shown="5" w233 {
          frame 0, Default {
            n287 = property on="Color Box 26" class="ColBox"("Value"=u32 16711686 ("Color Box")) -> ()  [unwired: 2 in, 2 out]
          }
          frame 1 {
            n288 = property on="Color Box 26" class="ColBox"("Value"=u32 15728450 ("Color Box")) -> ()  [unwired: 2 in, 2 out]
          }
          frame 2 {
            n289 = property on="Color Box 26" class="ColBox"("Value"=u32 16752640 ("Color Box")) -> ()  [unwired: 2 in, 2 out]
          }
          frame 3 {
            n290 = property on="Color Box 26" class="ColBox"("Value"=u32 16711422 ("Color Box")) -> ()  [unwired: 2 in, 2 out]
          }
          frame 4 {
            n291 = property on="Color Box 26" class="ColBox"("Value"=u32 1535 ("Color Box")) -> ()  [unwired: 2 in, 2 out]
          }
          frame 5 {
            n292 = property on="Color Box 26" class="ColBox"("Value"=u32 2621184 ("Color Box")) -> ()  [unwired: 2 in, 2 out]
          }
        }
        n293 = case shown="3" w231 {
          frame 0, Default {
            n294 = property on="Color Box 25" class="ColBox"("Value"=u32 16711686 ("Color Box")) -> ()  [unwired: 2 in, 2 out]
          }
          frame 1 {
            n295 = property on="Color Box 25" class="ColBox"("Value"=u32 15728450 ("Color Box")) -> ()  [unwired: 2 in, 2 out]
          }
          frame 2 {
            n296 = property on="Color Box 25" class="ColBox"("Value"=u32 16752640 ("Color Box")) -> ()  [unwired: 2 in, 2 out]
          }
          frame 3 {
            n297 = property on="Color Box 25" class="ColBox"("Value"=u32 16711422 ("Color Box")) -> ()  [unwired: 2 in, 2 out]
          }
          frame 4 {
            n298 = property on="Color Box 25" class="ColBox"("Value"=u32 1535 ("Color Box")) -> ()  [unwired: 2 in, 2 out]
          }
          frame 5 {
            n299 = property on="Color Box 25" class="ColBox"("Value"=u32 2621184 ("Color Box")) -> ()  [unwired: 2 in, 2 out]
          }
        }
        n300 = case shown="3" w224 {
          frame 0, Default {
            n301 = property on="Color Box 34" class="ColBox"("Value"=u32 16711686 ("Color Box")) -> ()  [unwired: 2 in, 2 out]
          }
          frame 1 {
            n302 = property on="Color Box 34" class="ColBox"("Value"=u32 15728450 ("Color Box")) -> ()  [unwired: 2 in, 2 out]
          }
          frame 2 {
            n303 = property on="Color Box 34" class="ColBox"("Value"=u32 16752640 ("Color Box")) -> ()  [unwired: 2 in, 2 out]
          }
          frame 3 {
            n304 = property on="Color Box 34" class="ColBox"("Value"=u32 16711422 ("Color Box")) -> ()  [unwired: 2 in, 2 out]
          }
          frame 4 {
            n305 = property on="Color Box 34" class="ColBox"("Value"=u32 1535 ("Color Box")) -> ()  [unwired: 2 in, 2 out]
          }
          frame 5 {
            n306 = property on="Color Box 34" class="ColBox"("Value"=u32 2621184 ("Color Box")) -> ()  [unwired: 2 in, 2 out]
          }
        }
        n307 = case shown="3" w226 {
          frame 0, Default {
            n308 = property on="Color Box 33" class="ColBox"("Value"=u32 16711686 ("Color Box")) -> ()  [unwired: 2 in, 2 out]
          }
          frame 1 {
            n309 = property on="Color Box 33" class="ColBox"("Value"=u32 15728450 ("Color Box")) -> ()  [unwired: 2 in, 2 out]
          }
          frame 2 {
            n310 = property on="Color Box 33" class="ColBox"("Value"=u32 16752640 ("Color Box")) -> ()  [unwired: 2 in, 2 out]
          }
          frame 3 {
            n311 = property on="Color Box 33" class="ColBox"("Value"=u32 16711422 ("Color Box")) -> ()  [unwired: 2 in, 2 out]
          }
          frame 4 {
            n312 = property on="Color Box 33" class="ColBox"("Value"=u32 1535 ("Color Box")) -> ()  [unwired: 2 in, 2 out]
          }
          frame 5 {
            n313 = property on="Color Box 33" class="ColBox"("Value"=u32 2621184 ("Color Box")) -> ()  [unwired: 2 in, 2 out]
          }
        }
        n314 = case shown="3" w137 {
          frame 0, Default {
            n315 = property on="Color Box 47" class="ColBox"("Value"=u32 16711686 ("Color Box")) -> ()  [unwired: 2 in, 2 out]
          }
          frame 1 {
            n316 = property on="Color Box 47" class="ColBox"("Value"=u32 15728450 ("Color Box")) -> ()  [unwired: 2 in, 2 out]
          }
          frame 2 {
            n317 = property on="Color Box 47" class="ColBox"("Value"=u32 16752640 ("Color Box")) -> ()  [unwired: 2 in, 2 out]
          }
          frame 3 {
            n318 = property on="Color Box 47" class="ColBox"("Value"=u32 16711422 ("Color Box")) -> ()  [unwired: 2 in, 2 out]
          }
          frame 4 {
            n319 = property on="Color Box 47" class="ColBox"("Value"=u32 1535 ("Color Box")) -> ()  [unwired: 2 in, 2 out]
          }
          frame 5 {
            n320 = property on="Color Box 47" class="ColBox"("Value"=u32 2621184 ("Color Box")) -> ()  [unwired: 2 in, 2 out]
          }
        }
        n321 = case shown="3" w135 {
          frame 0, Default {
            n322 = property on="Color Box 48" class="ColBox"("Value"=u32 16711686 ("Color Box")) -> ()  [unwired: 2 in, 2 out]
          }
          frame 1 {
            n323 = property on="Color Box 48" class="ColBox"("Value"=u32 15728450 ("Color Box")) -> ()  [unwired: 2 in, 2 out]
          }
          frame 2 {
            n324 = property on="Color Box 48" class="ColBox"("Value"=u32 16752640 ("Color Box")) -> ()  [unwired: 2 in, 2 out]
          }
          frame 3 {
            n325 = property on="Color Box 48" class="ColBox"("Value"=u32 16711422 ("Color Box")) -> ()  [unwired: 2 in, 2 out]
          }
          frame 4 {
            n326 = property on="Color Box 48" class="ColBox"("Value"=u32 1535 ("Color Box")) -> ()  [unwired: 2 in, 2 out]
          }
          frame 5 {
            n327 = property on="Color Box 48" class="ColBox"("Value"=u32 2621184 ("Color Box")) -> ()  [unwired: 2 in, 2 out]
          }
        }
        n328 = case shown="3" w345 {
          frame 0, Default {
            n329 = property on="Color Box 9" class="ColBox"("Value"=u32 16711686 ("Color Box")) -> ()  [unwired: 2 in, 2 out]
          }
          frame 1 {
            n330 = property on="Color Box 9" class="ColBox"("Value"=u32 15728450 ("Color Box")) -> ()  [unwired: 2 in, 2 out]
          }
          frame 2 {
            n331 = property on="Color Box 9" class="ColBox"("Value"=u32 16752640 ("Color Box")) -> ()  [unwired: 2 in, 2 out]
          }
          frame 3 {
            n332 = property on="Color Box 9" class="ColBox"("Value"=u32 16711422 ("Color Box")) -> ()  [unwired: 2 in, 2 out]
          }
          frame 4 {
            n333 = property on="Color Box 9" class="ColBox"("Value"=u32 1535 ("Color Box")) -> ()  [unwired: 2 in, 2 out]
          }
          frame 5 {
            n334 = property on="Color Box 9" class="ColBox"("Value"=u32 2621184 ("Color Box")) -> ()  [unwired: 2 in, 2 out]
          }
        }
        n335 = case shown="3" w343 {
          frame 0, Default {
            n336 = property on="Color Box 10" class="ColBox"("Value"=u32 16711686 ("Color Box")) -> ()  [unwired: 2 in, 2 out]
          }
          frame 1 {
            n337 = property on="Color Box 10" class="ColBox"("Value"=u32 15728450 ("Color Box")) -> ()  [unwired: 2 in, 2 out]
          }
          frame 2 {
            n338 = property on="Color Box 10" class="ColBox"("Value"=u32 16752640 ("Color Box")) -> ()  [unwired: 2 in, 2 out]
          }
          frame 3 {
            n339 = property on="Color Box 10" class="ColBox"("Value"=u32 16711422 ("Color Box")) -> ()  [unwired: 2 in, 2 out]
          }
          frame 4 {
            n340 = property on="Color Box 10" class="ColBox"("Value"=u32 1535 ("Color Box")) -> ()  [unwired: 2 in, 2 out]
          }
          frame 5 {
            n341 = property on="Color Box 10" class="ColBox"("Value"=u32 2621184 ("Color Box")) -> ()  [unwired: 2 in, 2 out]
          }
        }
        n342 = case shown="3" w288 {
          frame 0, Default {
            n343 = property on="Color Box 17" class="ColBox"("Value"=u32 16711686 ("Color Box")) -> ()  [unwired: 2 in, 2 out]
          }
          frame 1 {
            n344 = property on="Color Box 17" class="ColBox"("Value"=u32 15728450 ("Color Box")) -> ()  [unwired: 2 in, 2 out]
          }
          frame 2 {
            n345 = property on="Color Box 17" class="ColBox"("Value"=u32 16752640 ("Color Box")) -> ()  [unwired: 2 in, 2 out]
          }
          frame 3 {
            n346 = property on="Color Box 17" class="ColBox"("Value"=u32 16711422 ("Color Box")) -> ()  [unwired: 2 in, 2 out]
          }
          frame 4 {
            n347 = property on="Color Box 17" class="ColBox"("Value"=u32 1535 ("Color Box")) -> ()  [unwired: 2 in, 2 out]
          }
          frame 5 {
            n348 = property on="Color Box 17" class="ColBox"("Value"=u32 2621184 ("Color Box")) -> ()  [unwired: 2 in, 2 out]
          }
        }
        n349 = case shown="3" w290 {
          frame 0, Default {
            n350 = property on="Color Box 18" class="ColBox"("Value"=u32 16711686 ("Color Box")) -> ()  [unwired: 2 in, 2 out]
          }
          frame 1 {
            n351 = property on="Color Box 18" class="ColBox"("Value"=u32 15728450 ("Color Box")) -> ()  [unwired: 2 in, 2 out]
          }
          frame 2 {
            n352 = property on="Color Box 18" class="ColBox"("Value"=u32 16752640 ("Color Box")) -> ()  [unwired: 2 in, 2 out]
          }
          frame 3 {
            n353 = property on="Color Box 18" class="ColBox"("Value"=u32 16711422 ("Color Box")) -> ()  [unwired: 2 in, 2 out]
          }
          frame 4 {
            n354 = property on="Color Box 18" class="ColBox"("Value"=u32 1535 ("Color Box")) -> ()  [unwired: 2 in, 2 out]
          }
          frame 5 {
            n355 = property on="Color Box 18" class="ColBox"("Value"=u32 2621184 ("Color Box")) -> ()  [unwired: 2 in, 2 out]
          }
        }
        n356 = case shown="3" w336 {
          frame 0, Default {
            n357 = property on="Color Box 13" class="ColBox"("Value"=u32 16711686 ("Color Box")) -> ()  [unwired: 2 in, 2 out]
          }
          frame 1 {
            n358 = property on="Color Box 13" class="ColBox"("Value"=u32 15728450 ("Color Box")) -> ()  [unwired: 2 in, 2 out]
          }
          frame 2 {
            n359 = property on="Color Box 13" class="ColBox"("Value"=u32 16752640 ("Color Box")) -> ()  [unwired: 2 in, 2 out]
          }
          frame 3 {
            n360 = property on="Color Box 13" class="ColBox"("Value"=u32 16711422 ("Color Box")) -> ()  [unwired: 2 in, 2 out]
          }
          frame 4 {
            n361 = property on="Color Box 13" class="ColBox"("Value"=u32 1535 ("Color Box")) -> ()  [unwired: 2 in, 2 out]
          }
          frame 5 {
            n362 = property on="Color Box 13" class="ColBox"("Value"=u32 2621184 ("Color Box")) -> ()  [unwired: 2 in, 2 out]
          }
        }
        n363 = case shown="3" w338 {
          frame 0, Default {
            n364 = property on="Color Box 14" class="ColBox"("Value"=u32 16711686 ("Color Box")) -> ()  [unwired: 2 in, 2 out]
          }
          frame 1 {
            n365 = property on="Color Box 14" class="ColBox"("Value"=u32 15728450 ("Color Box")) -> ()  [unwired: 2 in, 2 out]
          }
          frame 2 {
            n366 = property on="Color Box 14" class="ColBox"("Value"=u32 16752640 ("Color Box")) -> ()  [unwired: 2 in, 2 out]
          }
          frame 3 {
            n367 = property on="Color Box 14" class="ColBox"("Value"=u32 16711422 ("Color Box")) -> ()  [unwired: 2 in, 2 out]
          }
          frame 4 {
            n368 = property on="Color Box 14" class="ColBox"("Value"=u32 1535 ("Color Box")) -> ()  [unwired: 2 in, 2 out]
          }
          frame 5 {
            n369 = property on="Color Box 14" class="ColBox"("Value"=u32 2621184 ("Color Box")) -> ()  [unwired: 2 in, 2 out]
          }
        }
        n370 = case shown="3" w297 {
          frame 0, Default {
            n371 = property on="Color Box 21" class="ColBox"("Value"=u32 16711686 ("Color Box")) -> ()  [unwired: 2 in, 2 out]
          }
          frame 1 {
            n372 = property on="Color Box 21" class="ColBox"("Value"=u32 15728450 ("Color Box")) -> ()  [unwired: 2 in, 2 out]
          }
          frame 2 {
            n373 = property on="Color Box 21" class="ColBox"("Value"=u32 16752640 ("Color Box")) -> ()  [unwired: 2 in, 2 out]
          }
          frame 3 {
            n374 = property on="Color Box 21" class="ColBox"("Value"=u32 16711422 ("Color Box")) -> ()  [unwired: 2 in, 2 out]
          }
          frame 4 {
            n375 = property on="Color Box 21" class="ColBox"("Value"=u32 1535 ("Color Box")) -> ()  [unwired: 2 in, 2 out]
          }
          frame 5 {
            n376 = property on="Color Box 21" class="ColBox"("Value"=u32 2621184 ("Color Box")) -> ()  [unwired: 2 in, 2 out]
          }
        }
        n377 = case shown="3" w295 {
          frame 0, Default {
            n378 = property on="Color Box 22" class="ColBox"("Value"=u32 16711686 ("Color Box")) -> ()  [unwired: 2 in, 2 out]
          }
          frame 1 {
            n379 = property on="Color Box 22" class="ColBox"("Value"=u32 15728450 ("Color Box")) -> ()  [unwired: 2 in, 2 out]
          }
          frame 2 {
            n380 = property on="Color Box 22" class="ColBox"("Value"=u32 16752640 ("Color Box")) -> ()  [unwired: 2 in, 2 out]
          }
          frame 3 {
            n381 = property on="Color Box 22" class="ColBox"("Value"=u32 16711422 ("Color Box")) -> ()  [unwired: 2 in, 2 out]
          }
          frame 4 {
            n382 = property on="Color Box 22" class="ColBox"("Value"=u32 1535 ("Color Box")) -> ()  [unwired: 2 in, 2 out]
          }
          frame 5 {
            n383 = property on="Color Box 22" class="ColBox"("Value"=u32 2621184 ("Color Box")) -> ()  [unwired: 2 in, 2 out]
          }
        }
        n384 = case shown="3" w352 {
          frame 0, Default {
            n385 = property on="Color Box 11" class="ColBox"("Value"=u32 16711686 ("Color Box")) -> ()  [unwired: 2 in, 2 out]
          }
          frame 1 {
            n386 = property on="Color Box 11" class="ColBox"("Value"=u32 15728450 ("Color Box")) -> ()  [unwired: 2 in, 2 out]
          }
          frame 2 {
            n387 = property on="Color Box 11" class="ColBox"("Value"=u32 16752640 ("Color Box")) -> ()  [unwired: 2 in, 2 out]
          }
          frame 3 {
            n388 = property on="Color Box 11" class="ColBox"("Value"=u32 16711422 ("Color Box")) -> ()  [unwired: 2 in, 2 out]
          }
          frame 4 {
            n389 = property on="Color Box 11" class="ColBox"("Value"=u32 1535 ("Color Box")) -> ()  [unwired: 2 in, 2 out]
          }
          frame 5 {
            n390 = property on="Color Box 11" class="ColBox"("Value"=u32 2621184 ("Color Box")) -> ()  [unwired: 2 in, 2 out]
          }
        }
        n391 = case shown="3" w354 {
          frame 0, Default {
            n392 = property on="Color Box 12" class="ColBox"("Value"=u32 16711686 ("Color Box")) -> ()  [unwired: 2 in, 2 out]
          }
          frame 1 {
            n393 = property on="Color Box 12" class="ColBox"("Value"=u32 15728450 ("Color Box")) -> ()  [unwired: 2 in, 2 out]
          }
          frame 2 {
            n394 = property on="Color Box 12" class="ColBox"("Value"=u32 16752640 ("Color Box")) -> ()  [unwired: 2 in, 2 out]
          }
          frame 3 {
            n395 = property on="Color Box 12" class="ColBox"("Value"=u32 16711422 ("Color Box")) -> ()  [unwired: 2 in, 2 out]
          }
          frame 4 {
            n396 = property on="Color Box 12" class="ColBox"("Value"=u32 1535 ("Color Box")) -> ()  [unwired: 2 in, 2 out]
          }
          frame 5 {
            n397 = property on="Color Box 12" class="ColBox"("Value"=u32 2621184 ("Color Box")) -> ()  [unwired: 2 in, 2 out]
          }
        }
        n398 = case shown="3" w281 {
          frame 0, Default {
            n399 = property on="Color Box 19" class="ColBox"("Value"=u32 16711686 ("Color Box")) -> ()  [unwired: 2 in, 2 out]
          }
          frame 1 {
            n400 = property on="Color Box 19" class="ColBox"("Value"=u32 15728450 ("Color Box")) -> ()  [unwired: 2 in, 2 out]
          }
          frame 2 {
            n401 = property on="Color Box 19" class="ColBox"("Value"=u32 16752640 ("Color Box")) -> ()  [unwired: 2 in, 2 out]
          }
          frame 3 {
            n402 = property on="Color Box 19" class="ColBox"("Value"=u32 16711422 ("Color Box")) -> ()  [unwired: 2 in, 2 out]
          }
          frame 4 {
            n403 = property on="Color Box 19" class="ColBox"("Value"=u32 1535 ("Color Box")) -> ()  [unwired: 2 in, 2 out]
          }
          frame 5 {
            n404 = property on="Color Box 19" class="ColBox"("Value"=u32 2621184 ("Color Box")) -> ()  [unwired: 2 in, 2 out]
          }
        }
        n405 = case shown="3" w279 {
          frame 0, Default {
            n406 = property on="Color Box 20" class="ColBox"("Value"=u32 16711686 ("Color Box")) -> ()  [unwired: 2 in, 2 out]
          }
          frame 1 {
            n407 = property on="Color Box 20" class="ColBox"("Value"=u32 15728450 ("Color Box")) -> ()  [unwired: 2 in, 2 out]
          }
          frame 2 {
            n408 = property on="Color Box 20" class="ColBox"("Value"=u32 16752640 ("Color Box")) -> ()  [unwired: 2 in, 2 out]
          }
          frame 3 {
            n409 = property on="Color Box 20" class="ColBox"("Value"=u32 16711422 ("Color Box")) -> ()  [unwired: 2 in, 2 out]
          }
          frame 4 {
            n410 = property on="Color Box 20" class="ColBox"("Value"=u32 1535 ("Color Box")) -> ()  [unwired: 2 in, 2 out]
          }
          frame 5 {
            n411 = property on="Color Box 20" class="ColBox"("Value"=u32 2621184 ("Color Box")) -> ()  [unwired: 2 in, 2 out]
          }
        }
        n412 = case shown="3" w376 {
          frame 0, Default {
            n413 = property on="Color Box 5" class="ColBox"("Value"=u32 16711686 ("Color Box")) -> ()  [unwired: 2 in, 2 out]
          }
          frame 1 {
            n414 = property on="Color Box 5" class="ColBox"("Value"=u32 15728450 ("Color Box")) -> ()  [unwired: 2 in, 2 out]
          }
          frame 2 {
            n415 = property on="Color Box 5" class="ColBox"("Value"=u32 16752640 ("Color Box")) -> ()  [unwired: 2 in, 2 out]
          }
          frame 3 {
            n416 = property on="Color Box 5" class="ColBox"("Value"=u32 16711422 ("Color Box")) -> ()  [unwired: 2 in, 2 out]
          }
          frame 4 {
            n417 = property on="Color Box 5" class="ColBox"("Value"=u32 1535 ("Color Box")) -> ()  [unwired: 2 in, 2 out]
          }
          frame 5 {
            n418 = property on="Color Box 5" class="ColBox"("Value"=u32 2621184 ("Color Box")) -> ()  [unwired: 2 in, 2 out]
          }
        }
        n419 = case shown="3" w378 {
          frame 0, Default {
            n420 = property on="Color Box 6" class="ColBox"("Value"=u32 16711686 ("Color Box")) -> ()  [unwired: 2 in, 2 out]
          }
          frame 1 {
            n421 = property on="Color Box 6" class="ColBox"("Value"=u32 15728450 ("Color Box")) -> ()  [unwired: 2 in, 2 out]
          }
          frame 2 {
            n422 = property on="Color Box 6" class="ColBox"("Value"=u32 16752640 ("Color Box")) -> ()  [unwired: 2 in, 2 out]
          }
          frame 3 {
            n423 = property on="Color Box 6" class="ColBox"("Value"=u32 16711422 ("Color Box")) -> ()  [unwired: 2 in, 2 out]
          }
          frame 4 {
            n424 = property on="Color Box 6" class="ColBox"("Value"=u32 1535 ("Color Box")) -> ()  [unwired: 2 in, 2 out]
          }
          frame 5 {
            n425 = property on="Color Box 6" class="ColBox"("Value"=u32 2621184 ("Color Box")) -> ()  [unwired: 2 in, 2 out]
          }
        }
        n426 = case shown="2" w329 {
          frame 0, Default {
            n427 = property on="Color Box 15" class="ColBox"("Value"=u32 16711686 ("Color Box")) -> ()  [unwired: 2 in, 2 out]
          }
          frame 1 {
            n428 = property on="Color Box 15" class="ColBox"("Value"=u32 15728450 ("Color Box")) -> ()  [unwired: 2 in, 2 out]
          }
          frame 2 {
            n429 = property on="Color Box 15" class="ColBox"("Value"=u32 16752640 ("Color Box")) -> ()  [unwired: 2 in, 2 out]
          }
          frame 3 {
            n430 = property on="Color Box 15" class="ColBox"("Value"=u32 16711422 ("Color Box")) -> ()  [unwired: 2 in, 2 out]
          }
          frame 4 {
            n431 = property on="Color Box 15" class="ColBox"("Value"=u32 1535 ("Color Box")) -> ()  [unwired: 2 in, 2 out]
          }
          frame 5 {
            n432 = property on="Color Box 15" class="ColBox"("Value"=u32 2621184 ("Color Box")) -> ()  [unwired: 2 in, 2 out]
          }
        }
        n433 = case shown="3" w327 {
          frame 0, Default {
            n434 = property on="Color Box 16" class="ColBox"("Value"=u32 16711686 ("Color Box")) -> ()  [unwired: 2 in, 2 out]
          }
          frame 1 {
            n435 = property on="Color Box 16" class="ColBox"("Value"=u32 15728450 ("Color Box")) -> ()  [unwired: 2 in, 2 out]
          }
          frame 2 {
            n436 = property on="Color Box 16" class="ColBox"("Value"=u32 16752640 ("Color Box")) -> ()  [unwired: 2 in, 2 out]
          }
          frame 3 {
            n437 = property on="Color Box 16" class="ColBox"("Value"=u32 16711422 ("Color Box")) -> ()  [unwired: 2 in, 2 out]
          }
          frame 4 {
            n438 = property on="Color Box 16" class="ColBox"("Value"=u32 1535 ("Color Box")) -> ()  [unwired: 2 in, 2 out]
          }
          frame 5 {
            n439 = property on="Color Box 16" class="ColBox"("Value"=u32 2621184 ("Color Box")) -> ()  [unwired: 2 in, 2 out]
          }
        }
        n440 = case shown="1" w304 {
          frame 0, Default {
            n441 = property on="Color Box 23" class="ColBox"("Value"=u32 16711686 ("Color Box")) -> ()  [unwired: 2 in, 2 out]
          }
          frame 1 {
            n442 = property on="Color Box 23" class="ColBox"("Value"=u32 15728450 ("Color Box")) -> ()  [unwired: 2 in, 2 out]
          }
          frame 2 {
            n443 = property on="Color Box 23" class="ColBox"("Value"=u32 16752640 ("Color Box")) -> ()  [unwired: 2 in, 2 out]
          }
          frame 3 {
            n444 = property on="Color Box 23" class="ColBox"("Value"=u32 16711422 ("Color Box")) -> ()  [unwired: 2 in, 2 out]
          }
          frame 4 {
            n445 = property on="Color Box 23" class="ColBox"("Value"=u32 1535 ("Color Box")) -> ()  [unwired: 2 in, 2 out]
          }
          frame 5 {
            n446 = property on="Color Box 23" class="ColBox"("Value"=u32 2621184 ("Color Box")) -> ()  [unwired: 2 in, 2 out]
          }
        }
        n447 = case shown="3" w306 {
          frame 0, Default {
            n448 = property on="Color Box 24" class="ColBox"("Value"=u32 16711686 ("Color Box")) -> ()  [unwired: 2 in, 2 out]
          }
          frame 1 {
            n449 = property on="Color Box 24" class="ColBox"("Value"=u32 15728450 ("Color Box")) -> ()  [unwired: 2 in, 2 out]
          }
          frame 2 {
            n450 = property on="Color Box 24" class="ColBox"("Value"=u32 16752640 ("Color Box")) -> ()  [unwired: 2 in, 2 out]
          }
          frame 3 {
            n451 = property on="Color Box 24" class="ColBox"("Value"=u32 16711422 ("Color Box")) -> ()  [unwired: 2 in, 2 out]
          }
          frame 4 {
            n452 = property on="Color Box 24" class="ColBox"("Value"=u32 1535 ("Color Box")) -> ()  [unwired: 2 in, 2 out]
          }
          frame 5 {
            n453 = property on="Color Box 24" class="ColBox"("Value"=u32 2621184 ("Color Box")) -> ()  [unwired: 2 in, 2 out]
          }
        }
        n454 = case shown="3" w389 {
          frame 0, Default {
            n455 = property on="Color Box 3" class="ColBox"("Value"=u32 16711686 ("Color Box")) -> ()  [unwired: 2 in, 2 out]
          }
          frame 1 {
            n456 = property on="Color Box 3" class="ColBox"("Value"=u32 15728450 ("Color Box")) -> ()  [unwired: 2 in, 2 out]
          }
          frame 2 {
            n457 = property on="Color Box 3" class="ColBox"("Value"=u32 16752640 ("Color Box")) -> ()  [unwired: 2 in, 2 out]
          }
          frame 3 {
            n458 = property on="Color Box 3" class="ColBox"("Value"=u32 16711422 ("Color Box")) -> ()  [unwired: 2 in, 2 out]
          }
          frame 4 {
            n459 = property on="Color Box 3" class="ColBox"("Value"=u32 1535 ("Color Box")) -> ()  [unwired: 2 in, 2 out]
          }
          frame 5 {
            n460 = property on="Color Box 3" class="ColBox"("Value"=u32 2621184 ("Color Box")) -> ()  [unwired: 2 in, 2 out]
          }
        }
        n461 = case shown="3" w387 {
          frame 0, Default {
            n462 = property on="Color Box 4" class="ColBox"("Value"=u32 16711686 ("Color Box")) -> ()  [unwired: 2 in, 2 out]
          }
          frame 1 {
            n463 = property on="Color Box 4" class="ColBox"("Value"=u32 15728450 ("Color Box")) -> ()  [unwired: 2 in, 2 out]
          }
          frame 2 {
            n464 = property on="Color Box 4" class="ColBox"("Value"=u32 16752640 ("Color Box")) -> ()  [unwired: 2 in, 2 out]
          }
          frame 3 {
            n465 = property on="Color Box 4" class="ColBox"("Value"=u32 16711422 ("Color Box")) -> ()  [unwired: 2 in, 2 out]
          }
          frame 4 {
            n466 = property on="Color Box 4" class="ColBox"("Value"=u32 1535 ("Color Box")) -> ()  [unwired: 2 in, 2 out]
          }
          frame 5 {
            n467 = property on="Color Box 4" class="ColBox"("Value"=u32 2621184 ("Color Box")) -> ()  [unwired: 2 in, 2 out]
          }
        }
        n468 = case shown="3" w369 {
          frame 0, Default {
            n469 = property on="Color Box 7" class="ColBox"("Value"=u32 16711686 ("Color Box")) -> ()  [unwired: 2 in, 2 out]
          }
          frame 1 {
            n470 = property on="Color Box 7" class="ColBox"("Value"=u32 15728450 ("Color Box")) -> ()  [unwired: 2 in, 2 out]
          }
          frame 2 {
            n471 = property on="Color Box 7" class="ColBox"("Value"=u32 16752640 ("Color Box")) -> ()  [unwired: 2 in, 2 out]
          }
          frame 3 {
            n472 = property on="Color Box 7" class="ColBox"("Value"=u32 16711422 ("Color Box")) -> ()  [unwired: 2 in, 2 out]
          }
          frame 4 {
            n473 = property on="Color Box 7" class="ColBox"("Value"=u32 1535 ("Color Box")) -> ()  [unwired: 2 in, 2 out]
          }
          frame 5 {
            n474 = property on="Color Box 7" class="ColBox"("Value"=u32 2621184 ("Color Box")) -> ()  [unwired: 2 in, 2 out]
          }
        }
        n475 = case shown="3" w367 {
          frame 0, Default {
            n476 = property on="Color Box 8" class="ColBox"("Value"=u32 16711686 ("Color Box")) -> ()  [unwired: 2 in, 2 out]
          }
          frame 1 {
            n477 = property on="Color Box 8" class="ColBox"("Value"=u32 15728450 ("Color Box")) -> ()  [unwired: 2 in, 2 out]
          }
          frame 2 {
            n478 = property on="Color Box 8" class="ColBox"("Value"=u32 16752640 ("Color Box")) -> ()  [unwired: 2 in, 2 out]
          }
          frame 3 {
            n479 = property on="Color Box 8" class="ColBox"("Value"=u32 16711422 ("Color Box")) -> ()  [unwired: 2 in, 2 out]
          }
          frame 4 {
            n480 = property on="Color Box 8" class="ColBox"("Value"=u32 1535 ("Color Box")) -> ()  [unwired: 2 in, 2 out]
          }
          frame 5 {
            n481 = property on="Color Box 8" class="ColBox"("Value"=u32 2621184 ("Color Box")) -> ()  [unwired: 2 in, 2 out]
          }
        }
        n482 = case shown="0, Default" w399 {
          frame 0, Default {
            n483 = property on="Color Box 2" class="ColBox"("Value"=u32 16711686 ("Color Box")) -> ()  [unwired: 2 in, 2 out]
          }
          frame 1 {
            n484 = property on="Color Box 2" class="ColBox"("Value"=u32 15728450 ("Color Box")) -> ()  [unwired: 2 in, 2 out]
          }
          frame 2 {
            n485 = property on="Color Box 2" class="ColBox"("Value"=u32 16752640 ("Color Box")) -> ()  [unwired: 2 in, 2 out]
          }
          frame 3 {
            n486 = property on="Color Box 2" class="ColBox"("Value"=u32 16711422 ("Color Box")) -> ()  [unwired: 2 in, 2 out]
          }
          frame 4 {
            n487 = property on="Color Box 2" class="ColBox"("Value"=u32 1535 ("Color Box")) -> ()  [unwired: 2 in, 2 out]
          }
          frame 5 {
            n488 = property on="Color Box 2" class="ColBox"("Value"=u32 2621184 ("Color Box")) -> ()  [unwired: 2 in, 2 out]
          }
        }
        n489 = case shown="3" w401 {
          frame 0, Default {
            n490 = property on="Color Box" class="ColBox"("Value"=u32 16711686 ("Color Box")) -> ()  [unwired: 2 in, 2 out]
          }
          frame 1 {
            n491 = property on="Color Box" class="ColBox"("Value"=u32 15728450 ("Color Box")) -> ()  [unwired: 2 in, 2 out]
          }
          frame 2 {
            n492 = property on="Color Box" class="ColBox"("Value"=u32 16752640 ("Color Box")) -> ()  [unwired: 2 in, 2 out]
          }
          frame 3 {
            n493 = property on="Color Box" class="ColBox"("Value"=u32 16711422 ("Color Box")) -> ()  [unwired: 2 in, 2 out]
          }
          frame 4 {
            n494 = property on="Color Box" class="ColBox"("Value"=u32 1535 ("Color Box")) -> ()  [unwired: 2 in, 2 out]
          }
          frame 5 {
            n495 = property on="Color Box" class="ColBox"("Value"=u32 2621184 ("Color Box")) -> ()  [unwired: 2 in, 2 out]
          }
        }
      }
      n496 = disable-structure shown="Disabled" {
        frame Disabled {
          n497 = property on="Blanc" class="DigNum (strict)" props=["Value"]() -> ()  [unwired: 2 in, 3 out]
          n498 = property on="Jaune" class="DigNum (strict)" props=["Value"]() -> ()  [unwired: 2 in, 3 out]
          n499 = property on="Bleu" class="DigNum (strict)" props=["Value"]() -> ()  [unwired: 2 in, 3 out]
          n500 = property on="Orange" class="DigNum (strict)" props=["Value"]() -> ()  [unwired: 2 in, 3 out]
          n501 = property on="Vert" class="DigNum (strict)" props=["Value"]() -> ()  [unwired: 2 in, 3 out]
        }
        frame Enabled {
        }
      }
      n502 = Not(x=w66) -> (.not. x?=w65:bool)
    }
    frame #1 {
      n503 = case shown="False" w693 {
        tunnel: [i32[][] [[0, 0, 0, 0, 0, 0, 0, 0, 0], [0, 0, 0, 0, 0, 0, 0, 0, 0], [0, 0, 0, 0, 0, 0, 0, 0, 0], [0, 0, 0, 0, 0, 0, 0, 0, 0], [0, 0, 0, 0, 0, 0, 0, 0, 0], [0, 0, 0, 0, 0, 0, 0, 0, 0]] w804] -> w694
        frame False {
        }
        frame True {
          n504 = property on="Color Box 12" class="ColBox"() -> ("Value"=w791:u32)  [unwired: 2 in, 2 out]
          n505 = property on="Color Box 16" class="ColBox"() -> ("Value"=w787:u32)  [unwired: 2 in, 2 out]
          n506 = property on="Color Box 13" class="ColBox"() -> ("Value"=w788:u32)  [unwired: 2 in, 2 out]
          n507 = property on="Color Box 14" class="ColBox"() -> ("Value"=w789:u32)  [unwired: 2 in, 2 out]
          n508 = property on="Color Box 11" class="ColBox"() -> ("Value"=w790:u32)  [unwired: 2 in, 2 out]
          n509 = property on="Color Box 10" class="ColBox"() -> ("Value"=w793:u32)  [unwired: 2 in, 2 out]
          n510 = property on="Color Box 15" class="ColBox"() -> ("Value"=w786:u32)  [unwired: 2 in, 2 out]
          n511 = property on="Color Box 9" class="ColBox"() -> ("Value"=w792:u32)  [unwired: 2 in, 2 out]
          n512 = property on="Color Box 2" class="ColBox"() -> ("Value"=w803:u32)  [unwired: 2 in, 2 out]
          n513 = property on="Color Box 6" class="ColBox"() -> ("Value"=w797:u32)  [unwired: 2 in, 2 out]
          n514 = property on="Color Box" class="ColBox"() -> ("Value"=w802:u32)  [unwired: 2 in, 2 out]
          n515 = property on="Color Box 8" class="ColBox"() -> ("Value"=w798:u32)  [unwired: 2 in, 2 out]
          n516 = property on="Color Box 5" class="ColBox"() -> ("Value"=w796:u32)  [unwired: 2 in, 2 out]
          n517 = property on="Color Box 7" class="ColBox"() -> ("Value"=w799:u32)  [unwired: 2 in, 2 out]
          n518 = property on="Color Box 3" class="ColBox"() -> ("Value"=w801:u32)  [unwired: 2 in, 2 out]
          n519 = property on="Color Box 4" class="ColBox"() -> ("Value"=w800:u32)  [unwired: 2 in, 2 out]
          n520 = property on="Color Box 23" class="ColBox"() -> ("Value"=w784:u32)  [unwired: 2 in, 2 out]
          n521 = property on="Color Box 46" class="ColBox"() -> ("Value"=w754:u32)  [unwired: 2 in, 2 out]
          n522 = property on="Color Box 48" class="ColBox"() -> ("Value"=w756:u32)  [unwired: 2 in, 2 out]
          n523 = property on="Color Box 47" class="ColBox"() -> ("Value"=w757:u32)  [unwired: 2 in, 2 out]
          n524 = property on="Color Box 43" class="ColBox"() -> ("Value"=w753:u32)  [unwired: 2 in, 2 out]
          n525 = property on="Color Box 24" class="ColBox"() -> ("Value"=w783:u32)  [unwired: 2 in, 2 out]
          n526 = property on="Color Box 42" class="ColBox"() -> ("Value"=w750:u32)  [unwired: 2 in, 2 out]
          n527 = property on="Color Box 21" class="ColBox"() -> ("Value"=w782:u32)  [unwired: 2 in, 2 out]
          n528 = property on="Color Box 18" class="ColBox"() -> ("Value"=w777:u32)  [unwired: 2 in, 2 out]
          n529 = property on="Color Box 45" class="ColBox"() -> ("Value"=w755:u32)  [unwired: 2 in, 2 out]
          n530 = property on="Color Box 20" class="ColBox"() -> ("Value"=w779:u32)  [unwired: 2 in, 2 out]
          n531 = property on="Color Box 22" class="ColBox"() -> ("Value"=w781:u32)  [unwired: 2 in, 2 out]
          n532 = property on="Color Box 19" class="ColBox"() -> ("Value"=w780:u32)  [unwired: 2 in, 2 out]
          n533 = property on="Color Box 17" class="ColBox"() -> ("Value"=w778:u32)  [unwired: 2 in, 2 out]
          n534 = property on="Color Box 26" class="ColBox"() -> ("Value"=w775:u32)  [unwired: 2 in, 2 out]
          n535 = property on="Color Box 41" class="ColBox"() -> ("Value"=w751:u32)  [unwired: 2 in, 2 out]
          n536 = property on="Color Box 44" class="ColBox"() -> ("Value"=w752:u32)  [unwired: 2 in, 2 out]
          n537 = property on="Color Box 25" class="ColBox"() -> ("Value"=w774:u32)  [unwired: 2 in, 2 out]
          n538 = property on="Color Box 28" class="ColBox"() -> ("Value"=w773:u32)  [unwired: 2 in, 2 out]
          n539 = property on="Color Box 36" class="ColBox"() -> ("Value"=w764:u32)  [unwired: 2 in, 2 out]
          n540 = property on="Color Box 27" class="ColBox"() -> ("Value"=w772:u32)  [unwired: 2 in, 2 out]
          n541 = property on="Color Box 34" class="ColBox"() -> ("Value"=w766:u32)  [unwired: 2 in, 2 out]
          n542 = property on="Color Box 33" class="ColBox"() -> ("Value"=w765:u32)  [unwired: 2 in, 2 out]
          n543 = property on="Color Box 35" class="ColBox"() -> ("Value"=w763:u32)  [unwired: 2 in, 2 out]
          n544 = property on="Color Box 29" class="ColBox"() -> ("Value"=w770:u32)  [unwired: 2 in, 2 out]
          n545 = property on="Color Box 30" class="ColBox"() -> ("Value"=w771:u32)  [unwired: 2 in, 2 out]
          n546 = property on="Color Box 38" class="ColBox"() -> ("Value"=w762:u32)  [unwired: 2 in, 2 out]
          n547 = property on="Color Box 31" class="ColBox"() -> ("Value"=w768:u32)  [unwired: 2 in, 2 out]
          n548 = property on="Color Box 40" class="ColBox"() -> ("Value"=w760:u32)  [unwired: 2 in, 2 out]
          n549 = property on="Color Box 37" class="ColBox"() -> ("Value"=w761:u32)  [unwired: 2 in, 2 out]
          n550 = property on="Color Box 39" class="ColBox"() -> ("Value"=w759:u32)  [unwired: 2 in, 2 out]
          n551 = property on="Color Box 32" class="ColBox"() -> ("Value"=w769:u32)  [unwired: 2 in, 2 out]
          n552 = case shown="2621184" w802 {
            tunnel: [404 1 3 2 0 5 4] -> w749
            frame Default {
            }
            frame 16711686 {
            }
            frame 15728450 {
            }
            frame 16752640 {
            }
            frame 16711422 {
            }
            frame 1535 {
            }
            frame 2621184 {
            }
          }
          n553 = case shown="1535" w803 {
            tunnel: [404 1 3 2 0 5 4] -> w746
            frame Default {
            }
            frame 16711686 {
            }
            frame 15728450 {
            }
            frame 16752640 {
            }
            frame 16711422 {
            }
            frame 1535 {
            }
            frame 2621184 {
            }
          }
          n554 = case shown="2621184" w796 {
            tunnel: [404 1 3 2 0 5 4] -> w743
            frame Default {
            }
            frame 16711686 {
            }
            frame 15728450 {
            }
            frame 16752640 {
            }
            frame 16711422 {
            }
            frame 1535 {
            }
            frame 2621184 {
            }
          }
          n555 = case shown="2621184" w801 {
            tunnel: [404 1 3 2 0 5 4] -> w748
            frame Default {
            }
            frame 16711686 {
            }
            frame 15728450 {
            }
            frame 16752640 {
            }
            frame 16711422 {
            }
            frame 1535 {
            }
            frame 2621184 {
            }
          }
          n556 = case shown="2621184" w800 {
            tunnel: [404 1 3 2 0 5 4] -> w747
            frame Default {
            }
            frame 16711686 {
            }
            frame 15728450 {
            }
            frame 16752640 {
            }
            frame 16711422 {
            }
            frame 1535 {
            }
            frame 2621184 {
            }
          }
          n557 = case shown="2621184" w798 {
            tunnel: [404 1 3 2 0 5 4] -> w744
            frame Default {
            }
            frame 16711686 {
            }
            frame 15728450 {
            }
            frame 16752640 {
            }
            frame 16711422 {
            }
            frame 1535 {
            }
            frame 2621184 {
            }
          }
          n558 = case shown="2621184" w799 {
            tunnel: [404 1 3 2 0 5 4] -> w745
            frame Default {
            }
            frame 16711686 {
            }
            frame 15728450 {
            }
            frame 16752640 {
            }
            frame 16711422 {
            }
            frame 1535 {
            }
            frame 2621184 {
            }
          }
          n559 = case shown="2621184" w797 {
            tunnel: [404 1 3 2 0 5 4] -> w742
            frame Default {
            }
            frame 16711686 {
            }
            frame 15728450 {
            }
            frame 16752640 {
            }
            frame 16711422 {
            }
            frame 1535 {
            }
            frame 2621184 {
            }
          }
          n560 = case shown="2621184" w787 {
            tunnel: [404 1 3 2 0 5 4] -> w740
            frame Default {
            }
            frame 16711686 {
            }
            frame 15728450 {
            }
            frame 16752640 {
            }
            frame 16711422 {
            }
            frame 1535 {
            }
            frame 2621184 {
            }
          }
          n561 = case shown="1535" w786 {
            tunnel: [404 1 3 2 0 5 4] -> w741
            frame Default {
            }
            frame 16711686 {
            }
            frame 15728450 {
            }
            frame 16752640 {
            }
            frame 16711422 {
            }
            frame 1535 {
            }
            frame 2621184 {
            }
          }
          n562 = case shown="2621184" w792 {
            tunnel: [404 1 3 2 0 5 4] -> w735
            frame Default {
            }
            frame 16711686 {
            }
            frame 15728450 {
            }
            frame 16752640 {
            }
            frame 16711422 {
            }
            frame 1535 {
            }
            frame 2621184 {
            }
          }
          n563 = case shown="2621184" w788 {
            tunnel: [404 1 3 2 0 5 4] -> w739
            frame Default {
            }
            frame 16711686 {
            }
            frame 15728450 {
            }
            frame 16752640 {
            }
            frame 16711422 {
            }
            frame 1535 {
            }
            frame 2621184 {
            }
          }
          n564 = case shown="2621184" w789 {
            tunnel: [404 1 3 2 0 5 4] -> w738
            frame Default {
            }
            frame 16711686 {
            }
            frame 15728450 {
            }
            frame 16752640 {
            }
            frame 16711422 {
            }
            frame 1535 {
            }
            frame 2621184 {
            }
          }
          n565 = case shown="2621184" w783 {
            tunnel: [404 1 3 2 0 5 4] -> w732
            frame Default {
            }
            frame 16711686 {
            }
            frame 15728450 {
            }
            frame 16752640 {
            }
            frame 16711422 {
            }
            frame 1535 {
            }
            frame 2621184 {
            }
          }
          n566 = case shown="1535" w784 {
            tunnel: [404 1 3 2 0 5 4] -> w733
            frame Default {
            }
            frame 16711686 {
            }
            frame 15728450 {
            }
            frame 16752640 {
            }
            frame 16711422 {
            }
            frame 1535 {
            }
            frame 2621184 {
            }
          }
          n567 = case shown="2621184" w791 {
            tunnel: [404 1 3 2 0 5 4] -> w736
            frame Default {
            }
            frame 16711686 {
            }
            frame 15728450 {
            }
            frame 16752640 {
            }
            frame 16711422 {
            }
            frame 1535 {
            }
            frame 2621184 {
            }
          }
          n568 = case shown="2621184" w778 {
            tunnel: [404 1 3 2 0 5 4] -> w711
            frame Default {
            }
            frame 16711686 {
            }
            frame 15728450 {
            }
            frame 16752640 {
            }
            frame 16711422 {
            }
            frame 1535 {
            }
            frame 2621184 {
            }
          }
          n569 = case shown="2621184" w790 {
            tunnel: [404 1 3 2 0 5 4] -> w737
            frame Default {
            }
            frame 16711686 {
            }
            frame 15728450 {
            }
            frame 16752640 {
            }
            frame 16711422 {
            }
            frame 1535 {
            }
            frame 2621184 {
            }
          }
          n570 = case shown="2621184" w793 {
            tunnel: [404 1 3 2 0 5 4] -> w734
            frame Default {
            }
            frame 16711686 {
            }
            frame 15728450 {
            }
            frame 16752640 {
            }
            frame 16711422 {
            }
            frame 1535 {
            }
            frame 2621184 {
            }
          }
          n571 = case shown="2621184" w782 {
            tunnel: [404 1 3 2 0 5 4] -> w727
            frame Default {
            }
            frame 16711686 {
            }
            frame 15728450 {
            }
            frame 16752640 {
            }
            frame 16711422 {
            }
            frame 1535 {
            }
            frame 2621184 {
            }
          }
          n572 = case shown="2621184" w781 {
            tunnel: [404 1 3 2 0 5 4] -> w724
            frame Default {
            }
            frame 16711686 {
            }
            frame 15728450 {
            }
            frame 16752640 {
            }
            frame 16711422 {
            }
            frame 1535 {
            }
            frame 2621184 {
            }
          }
          n573 = case shown="2621184" w779 {
            tunnel: [404 1 3 2 0 5 4] -> w718
            frame Default {
            }
            frame 16711686 {
            }
            frame 15728450 {
            }
            frame 16752640 {
            }
            frame 16711422 {
            }
            frame 1535 {
            }
            frame 2621184 {
            }
          }
          n574 = case shown="2621184" w780 {
            tunnel: [404 1 3 2 0 5 4] -> w719
            frame Default {
            }
            frame 16711686 {
            }
            frame 15728450 {
            }
            frame 16752640 {
            }
            frame 16711422 {
            }
            frame 1535 {
            }
            frame 2621184 {
            }
          }
          n575 = case shown="2621184" w777 {
            tunnel: [404 1 3 2 0 5 4] -> w710
            frame Default {
            }
            frame 16711686 {
            }
            frame 15728450 {
            }
            frame 16752640 {
            }
            frame 16711422 {
            }
            frame 1535 {
            }
            frame 2621184 {
            }
          }
          n576 = case shown="2621184" w774 {
            tunnel: [404 1 3 2 0 5 4] -> w730
            frame Default {
            }
            frame 16711686 {
            }
            frame 15728450 {
            }
            frame 16752640 {
            }
            frame 16711422 {
            }
            frame 1535 {
            }
            frame 2621184 {
            }
          }
          n577 = case shown="1535" w775 {
            tunnel: [404 1 3 2 0 5 4] -> w729
            frame Default {
            }
            frame 16711686 {
            }
            frame 15728450 {
            }
            frame 16752640 {
            }
            frame 16711422 {
            }
            frame 1535 {
            }
            frame 2621184 {
            }
          }
          n578 = case shown="2621184" w769 {
            tunnel: [404 1 3 2 0 5 4] -> w713
            frame Default {
            }
            frame 16711686 {
            }
            frame 15728450 {
            }
            frame 16752640 {
            }
            frame 16711422 {
            }
            frame 1535 {
            }
            frame 2621184 {
            }
          }
          n579 = case shown="2621184" w773 {
            tunnel: [404 1 3 2 0 5 4] -> w726
            frame Default {
            }
            frame 16711686 {
            }
            frame 15728450 {
            }
            frame 16752640 {
            }
            frame 16711422 {
            }
            frame 1535 {
            }
            frame 2621184 {
            }
          }
          n580 = case shown="2621184" w772 {
            tunnel: [404 1 3 2 0 5 4] -> w723
            frame Default {
            }
            frame 16711686 {
            }
            frame 15728450 {
            }
            frame 16752640 {
            }
            frame 16711422 {
            }
            frame 1535 {
            }
            frame 2621184 {
            }
          }
          n581 = case shown="2621184" w765 {
            tunnel: [404 1 3 2 0 5 4] -> w708
            frame Default {
            }
            frame 16711686 {
            }
            frame 15728450 {
            }
            frame 16752640 {
            }
            frame 16711422 {
            }
            frame 1535 {
            }
            frame 2621184 {
            }
          }
          n582 = case shown="1535" w766 {
            tunnel: [404 1 3 2 0 5 4] -> w709
            frame Default {
            }
            frame 16711686 {
            }
            frame 15728450 {
            }
            frame 16752640 {
            }
            frame 16711422 {
            }
            frame 1535 {
            }
            frame 2621184 {
            }
          }
          n583 = case shown="2621184" w760 {
            tunnel: [404 1 3 2 0 5 4] -> w703
            frame Default {
            }
            frame 16711686 {
            }
            frame 15728450 {
            }
            frame 16752640 {
            }
            frame 16711422 {
            }
            frame 1535 {
            }
            frame 2621184 {
            }
          }
          n584 = case shown="2621184" w770 {
            tunnel: [404 1 3 2 0 5 4] -> w717
            frame Default {
            }
            frame 16711686 {
            }
            frame 15728450 {
            }
            frame 16752640 {
            }
            frame 16711422 {
            }
            frame 1535 {
            }
            frame 2621184 {
            }
          }
          n585 = case shown="2621184" w771 {
            tunnel: [404 1 3 2 0 5 4] -> w720
            frame Default {
            }
            frame 16711686 {
            }
            frame 15728450 {
            }
            frame 16752640 {
            }
            frame 16711422 {
            }
            frame 1535 {
            }
            frame 2621184 {
            }
          }
          n586 = case shown="2621184" w768 {
            tunnel: [404 1 3 2 0 5 4] -> w712
            frame Default {
            }
            frame 16711686 {
            }
            frame 15728450 {
            }
            frame 16752640 {
            }
            frame 16711422 {
            }
            frame 1535 {
            }
            frame 2621184 {
            }
          }
          n587 = case shown="2621184" w764 {
            tunnel: [404 1 3 2 0 5 4] -> w707
            frame Default {
            }
            frame 16711686 {
            }
            frame 15728450 {
            }
            frame 16752640 {
            }
            frame 16711422 {
            }
            frame 1535 {
            }
            frame 2621184 {
            }
          }
          n588 = case shown="2621184" w763 {
            tunnel: [404 1 3 2 0 5 4] -> w706
            frame Default {
            }
            frame 16711686 {
            }
            frame 15728450 {
            }
            frame 16752640 {
            }
            frame 16711422 {
            }
            frame 1535 {
            }
            frame 2621184 {
            }
          }
          n589 = case shown="2621184" w761 {
            tunnel: [404 1 3 2 0 5 4] -> w704
            frame Default {
            }
            frame 16711686 {
            }
            frame 15728450 {
            }
            frame 16752640 {
            }
            frame 16711422 {
            }
            frame 1535 {
            }
            frame 2621184 {
            }
          }
          n590 = case shown="2621184" w762 {
            tunnel: [404 1 3 2 0 5 4] -> w705
            frame Default {
            }
            frame 16711686 {
            }
            frame 15728450 {
            }
            frame 16752640 {
            }
            frame 16711422 {
            }
            frame 1535 {
            }
            frame 2621184 {
            }
          }
          n591 = case shown="2621184" w759 {
            tunnel: [404 1 3 2 0 5 4] -> w702
            frame Default {
            }
            frame 16711686 {
            }
            frame 15728450 {
            }
            frame 16752640 {
            }
            frame 16711422 {
            }
            frame 1535 {
            }
            frame 2621184 {
            }
          }
          n592 = case shown="2621184" w756 {
            tunnel: [404 1 3 2 0 5 4] -> w731
            frame Default {
            }
            frame 16711686 {
            }
            frame 15728450 {
            }
            frame 16752640 {
            }
            frame 16711422 {
            }
            frame 1535 {
            }
            frame 2621184 {
            }
          }
          n593 = case shown="1535" w757 {
            tunnel: [404 1 3 2 0 5 4] -> w728
            frame Default {
            }
            frame 16711686 {
            }
            frame 15728450 {
            }
            frame 16752640 {
            }
            frame 16711422 {
            }
            frame 1535 {
            }
            frame 2621184 {
            }
          }
          n594 = case shown="2621184" w751 {
            tunnel: [404 1 3 2 0 5 4] -> w715
            frame Default {
            }
            frame 16711686 {
            }
            frame 15728450 {
            }
            frame 16752640 {
            }
            frame 16711422 {
            }
            frame 1535 {
            }
            frame 2621184 {
            }
          }
          n595 = case shown="2621184" w755 {
            tunnel: [404 1 3 2 0 5 4] -> w725
            frame Default {
            }
            frame 16711686 {
            }
            frame 15728450 {
            }
            frame 16752640 {
            }
            frame 16711422 {
            }
            frame 1535 {
            }
            frame 2621184 {
            }
          }
          n596 = case shown="2621184" w754 {
            tunnel: [404 1 3 2 0 5 4] -> w722
            frame Default {
            }
            frame 16711686 {
            }
            frame 15728450 {
            }
            frame 16752640 {
            }
            frame 16711422 {
            }
            frame 1535 {
            }
            frame 2621184 {
            }
          }
          n597 = case shown="2621184" w752 {
            tunnel: [404 1 3 2 0 5 4] -> w716
            frame Default {
            }
            frame 16711686 {
            }
            frame 15728450 {
            }
            frame 16752640 {
            }
            frame 16711422 {
            }
            frame 1535 {
            }
            frame 2621184 {
            }
          }
          n598 = case shown="2621184" w753 {
            tunnel: [404 1 3 2 0 5 4] -> w721
            frame Default {
            }
            frame 16711686 {
            }
            frame 15728450 {
            }
            frame 16752640 {
            }
            frame 16711422 {
            }
            frame 1535 {
            }
            frame 2621184 {
            }
          }
          n599 = case shown="2621184" w750 {
            tunnel: [404 1 3 2 0 5 4] -> w714
            frame Default {
            }
            frame 16711686 {
            }
            frame 15728450 {
            }
            frame 16752640 {
            }
            frame 16711422 {
            }
            frame 1535 {
            }
            frame 2621184 {
            }
          }
          n600 = Build Array(w749, w747, w748, w746, 0 ("element"), w745, w744, w742, w743) -> (w699:i32[])
          n601 = Build Array(w740, w738, w739, w741, 1 ("element"), w737, w736, w734, w735) -> (w700:i32[])
          n602 = Build Array(w732, w724, w727, w733, 5 ("element"), w719, w718, w710, w711) -> (w701:i32[])
          n603 = Build Array(w730, w723, w726, w729, 3 ("element"), w720, w717, w712, w713) -> (w698:i32[])
          n604 = Build Array(w703, w702, w704, w705, 2 ("element"), w709, w707, w706, w708) -> (w697:i32[])
          n605 = Build Array(w731, w722, w725, w728, 4 ("element"), w721, w716, w714, w715) -> (w696:i32[])
          n606 = Build Array(w700, w701, w697, w696, w699, w698) -> (w804:i32[][])
        }
      }
    }
  }
  "Array" <- w2
